vi "总磷总氮通讯.vi"() -> ()   [LabVIEW 2022 SP3, in "斯坦道CODcr.lvlib"]
uses:
  <vilib>/Plasmionique/MB Master/MB_Master_Serial/MB_Master_Serial.lvclass
  C:/Program Files (x86)/National Instruments/LabVIEW 2022/vi.lib/Plasmionique/MB Master/MB_Master/MB_Master.lvclass
  <vilib>/Plasmionique/MB Master/MB_Master_TCP/MB_Master_TCP.lvclass
  <vilib>/Utility/config.llb/Write Key (Boolean).vi
  <vilib>/Utility/config.llb/Write Key (String).vi
  <vilib>/Plasmionique/MB Master/MB_Master/MB_Master.lvclass
  <vilib>/Utility/config.llb/NI_LVConfig.lvlib
  <vilib>/Plasmionique/MB Master/MB Master.lvlib
  <vilib>/ptbypt/NI_PtbyPt.lvlib
panel:
  out "启用":bool=TRUE
  out "氨氮状态告警区":u16[](array[numeric])
  out "氨氮测量数据区":u16[](array[numeric])
  out "COD测量数据区":u16[](array[numeric])
  out "COD状态告警区":u16[](array[numeric])
  out "总氮测量数据区":u16[](array[numeric])
  out "总氮状态告警区":u16[](array[numeric])
  out "总磷状态告警区":u16[](array[numeric])
  out "总磷测量数据区":u16[](array[numeric])
  out "状态告警区":T1 {"告警代码" items=["无告警", "缺试剂告警", "缺水样告警", "缺蒸馏水告警", "缺标液告警", "仪表漏液告警", "标定异常告警", "超量程告警", "加热异常", "低试剂预警", "超上限告警", "超下限告警", "仪表内部其他异常", "滴定异常告警", "电极异常告警", "量程切换告警", "参数设置告警", "PH电极电位异常", "电导率电极异常", "浊度光度异常", "溶解氧电极异常", "溶解氧光强异常", "温度异常告警", "PH异常告警", "溶解氧异常告警", "电导率异常告警", "浊度异常告警", "叶绿素异常告警", "藻密度异常告警", "蓝绿藻异常告警", "ORP异常告警", "氨氮异常告警", "清洁刷异常告警", "SD卡异常告警", "蓝牙异常告警", "Wifi异常告警", "流程异常告警"]; "故障代码" items=["无故障", "电机故障", "温度故障", "通讯故障", "滴定故障"]}
  out "测量数据区":T2 {"单位" items=["ug/L", "mg/L", "ppm", "mg/m3", "cm", "ppb", "ug/m3", "%", "nmol/mol", "umol/mol", "MPN/L", "MPN/100ml", "ng/m3", "NTU", "无量纲", "ms/cm", "us/cm", "℃", "mV", "万个/L"]}
  out "status":bool
  out "关键参数区":T3
  in  "读关键参数区":bool
  in  "读状态告警区":bool
  in  "读测量数据区":bool
  in  "站号":u16(ring) items=["总磷"=1, "氨氮"=3]
  in  "停止":bool
  in  "启动":bool
  in  "控制命令":u16(ring) items=["启动测量"=1, "标样核查"=2, "零点核查"=3, "跨度核查"=4, "空白测试"=5, "平行样测试"=6, "加标回收"=7, "空白校准"=8, "标样校准"=9, "初始化（清洗）"=10, "停止测试"=11, "仪器重启"=12, "校时"=13, "模式设置"=14, "测量间隔设置"=15]
  in  "控制命令参数":u16[](array[numeric]) format="%04xH"
  in  "VISA Resource":refnum<visa-resource-name>
  in  "启用模块":bool
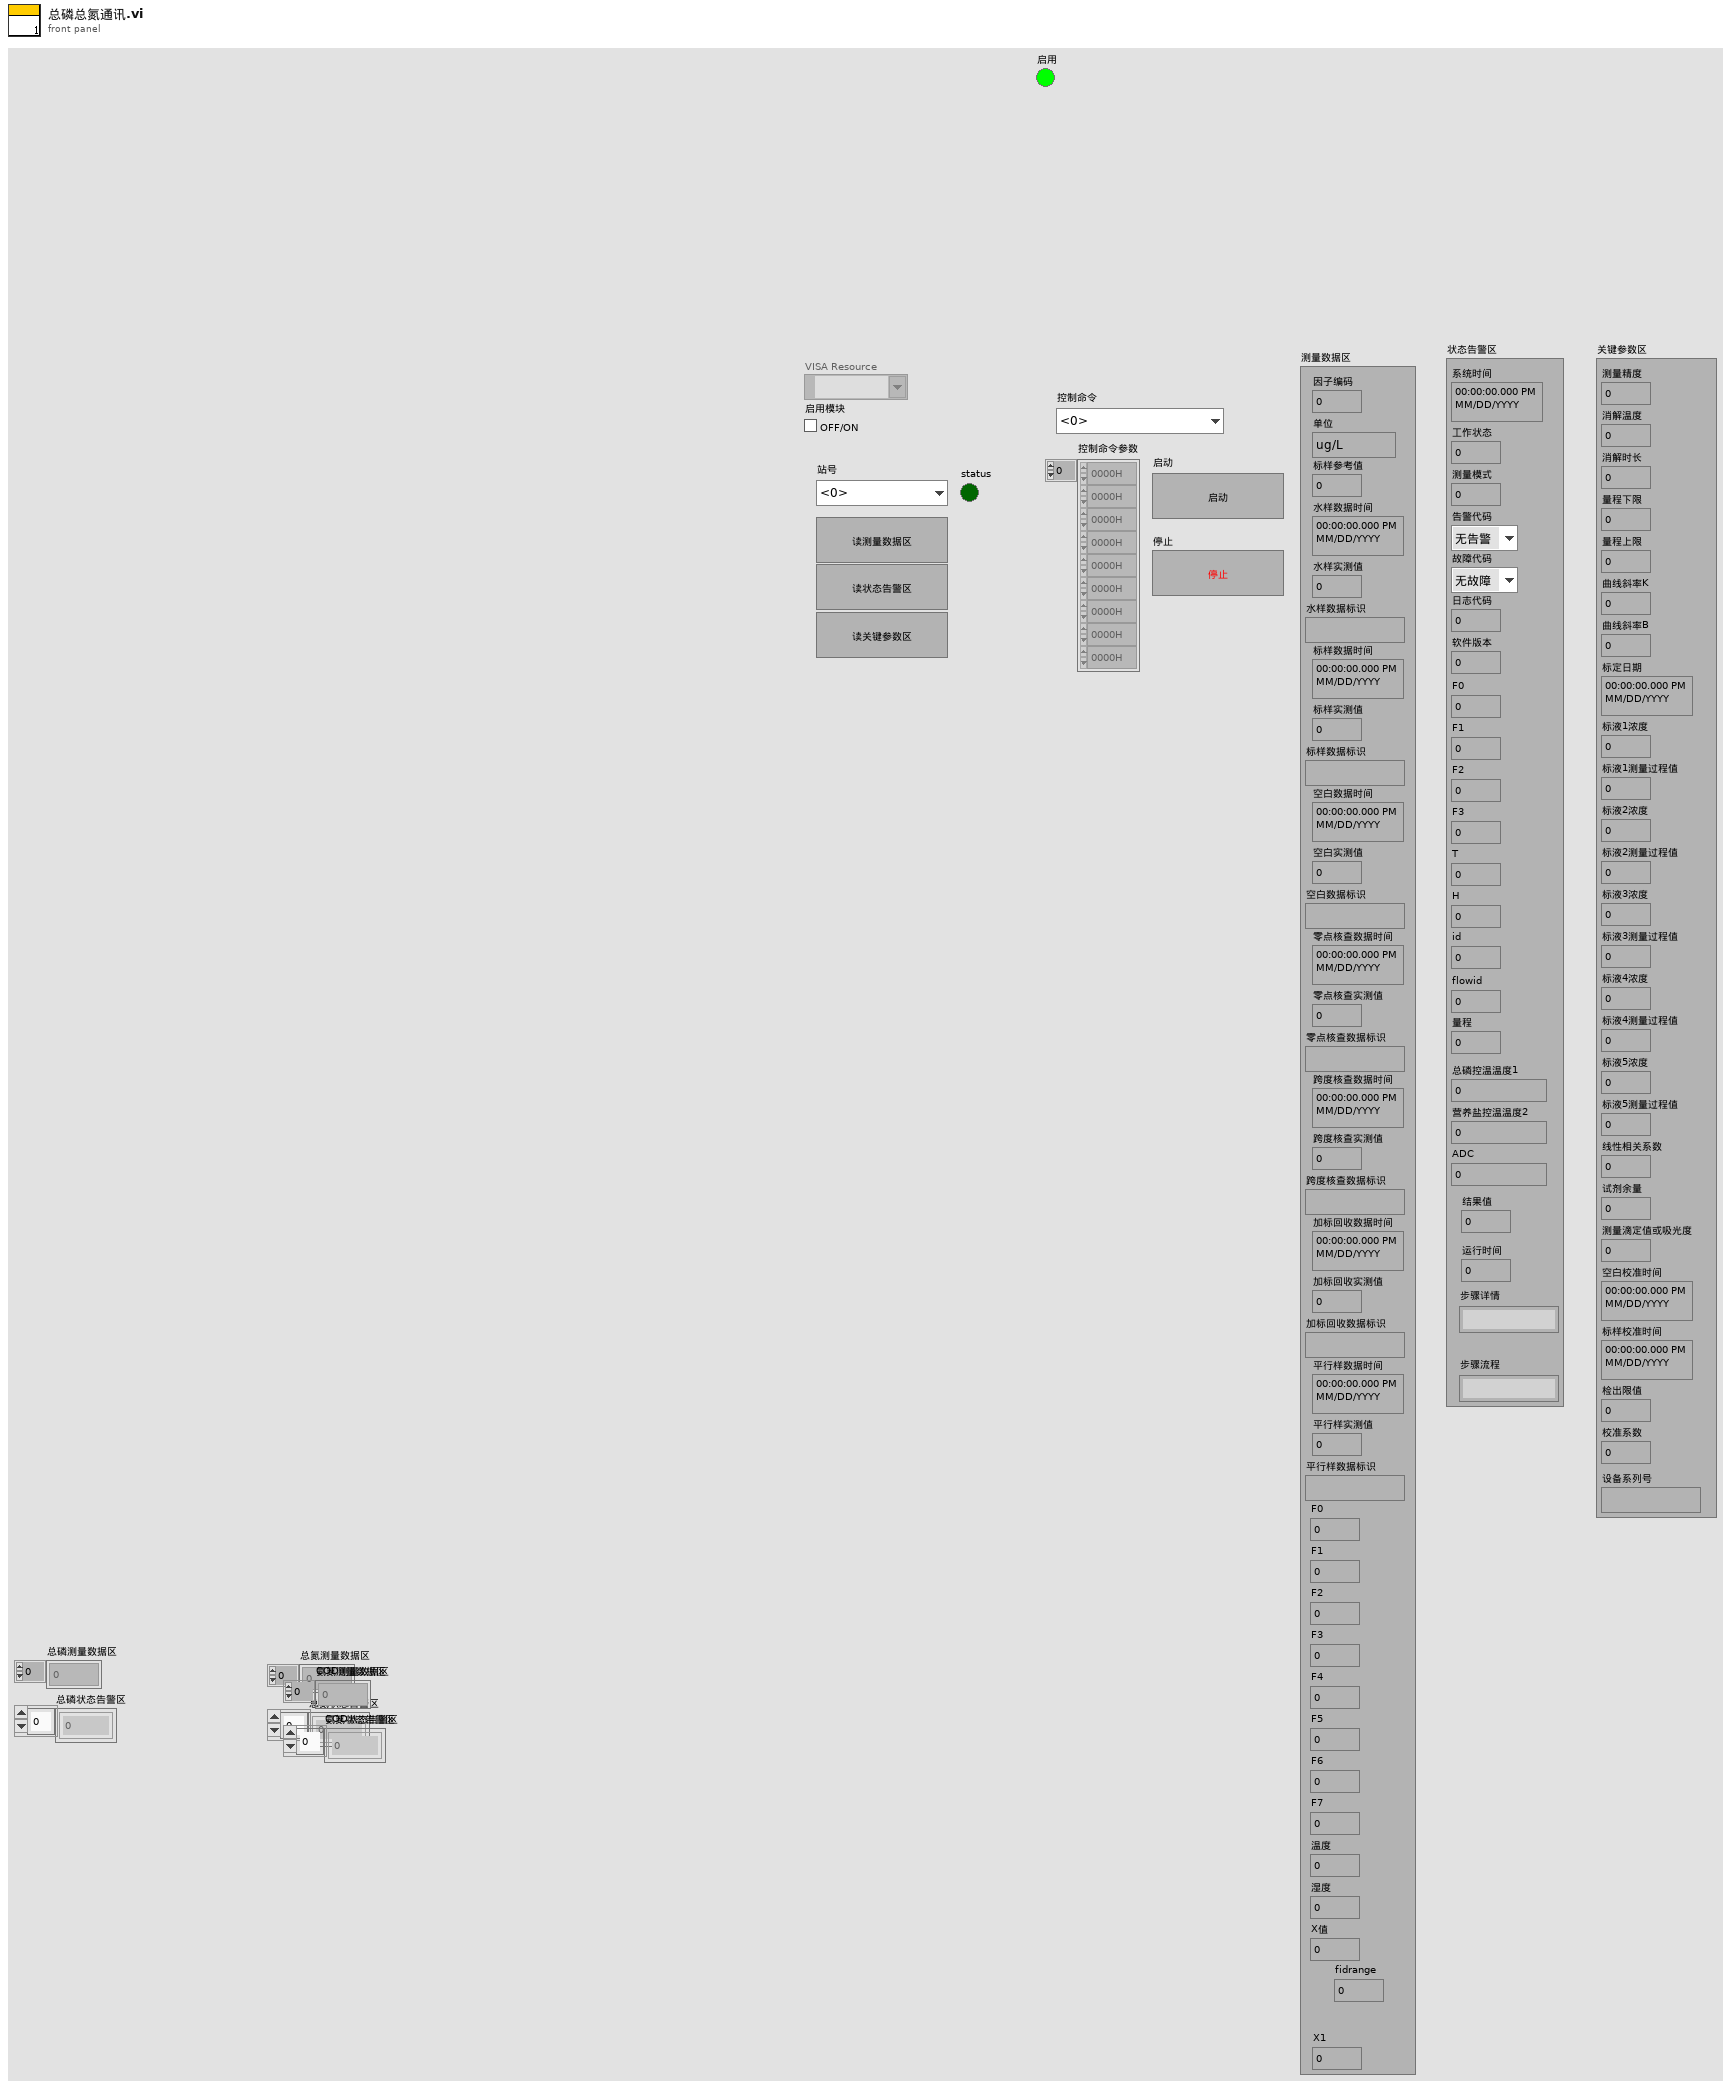
[diagram p1: front panel]
types:
  T1 = cluster{"系统时间":timestamp, "工作状态":u16, "测量模式":u16, "告警代码":u16, "故障代码":u16, "日志代码":u16, "软件版本":u16, "F0":sgl, "F1":sgl, "F2":sgl, "F3":sgl, "T":sgl, "H":sgl, "id":u16, "flowid":u16, "量程":u16, "总磷控温温度1":sgl, "营养盐控温温度2":sgl, "ADC":sgl, "结果值":sgl, "运行时间":u16, "步骤详情":string, "步骤流程":string}
  T2 = cluster{"因子编码":u32, "单位":u16, "标样参考值":sgl, "水样数据时间":timestamp, "水样实测值":sgl, "水样数据标识":string, "标样数据时间":timestamp, "标样实测值":sgl, "标样数据标识":string, "空白数据时间":timestamp, "空白实测值":sgl, "空白数据标识":string, "零点核查数据时间":timestamp, "零点核查实测值":sgl, "零点核查数据标识":string, "跨度核查数据时间":timestamp, "跨度核查实测值":sgl, "跨度核查数据标识":string, "加标回收数据时间":timestamp, "加标回收实测值":sgl, "加标回收数据标识":string, "平行样数据时间":timestamp, "平行样实测值":sgl, "平行样数据标识":string, "F0":sgl, "F1":sgl, "F2":sgl, "F3":sgl, "F4":sgl, "F5":sgl, "F6":sgl, "F7":sgl, "温度":sgl, "湿度":sgl, "X值":sgl, "fidrange":u16, "X1":sgl}
  T3 = cluster{"测量精度":u16, "消解温度":u16, "消解时长":u16, "量程下限":sgl, "量程上限":sgl, "曲线斜率K":sgl, "曲线斜率B":sgl, "标定日期":timestamp, "标液1浓度":sgl, "标液1测量过程值":sgl, "标液2浓度":sgl, "标液2测量过程值":sgl, "标液3浓度":sgl, "标液3测量过程值":sgl, "标液4浓度":sgl, "标液4测量过程值":sgl, "标液5浓度":sgl, "标液5测量过程值":sgl, "线性相关系数":sgl, "试剂余量":u32, "测量滴定值或吸光度":sgl, "空白校准时间":timestamp, "标样校准时间":timestamp, "检出限值":sgl, "校准系数":sgl, "设备系列号":string}
  T4 = cluster{"系统时间":timestamp, "工作状态":u16, "测量模式":enum16{"待机", "连续模式", "周期模式", "定点模式", "受控模式", "手动模式"}, "告警代码":u16, "故障代码":u16, "日志代码":u16, "软件版本":u16, "F0":sgl, "F1":sgl, "F2":sgl, "F3":sgl, "T":sgl, "H":sgl, "id":u16, "flowid":u16, "量程":u16, "总磷控温温度1":sgl, "营养盐控温温度2":sgl, "ADC":sgl}
  T5 = cluster{"因子编码":u32, "单位":u16, "标样参考值":sgl, "水样数据时间":timestamp, "水样实测值":sgl, "水样数据标识":string, "标样数据时间":timestamp, "标样实测值":sgl, "标样数据标识":string, "空白数据时间":timestamp, "空白实测值":sgl, "空白数据标识":string, "零点核查数据时间":timestamp, "零点核查实测值":sgl, "零点核查数据标识":string, "跨度核查数据时间":timestamp, "跨度核查实测值":sgl, "跨度核查数据标识":string, "加标回收数据时间":timestamp, "加标回收实测值":sgl, "加标回收数据标识":string, "平行样数据时间":timestamp, "平行样实测值":sgl, "平行样数据标识":string, "F0":sgl, "F1":sgl, "F2":sgl, "F3":sgl, "F4":sgl, "F5":sgl, "F6":sgl, "F7":sgl, "温度":sgl, "湿度":sgl, "X值":sgl, "fidrange":u16, "X1值":sgl}
  T6 = cluster{"测量精度":u16, "消解温度":u16, "消解时长":u16, "量程下限":sgl, "量程上限":sgl, "曲线斜率K":sgl, "曲线斜率B":sgl, "标定日期":timestamp, "标液1浓度":sgl, "标液1测量过程值":sgl, "标液2浓度":sgl, "标液2测量过程值":sgl, "标液3浓度":sgl, "标液3测量过程值":sgl, "标液4浓度":sgl, "标液4测量过程值":sgl, "标液5浓度":sgl, "标液5测量过程值":sgl, "线性相关系数":sgl, "试剂余量":u32, "测量滴定值或吸光度":sgl, "空白校准时间":timestamp, "标样校准时间":timestamp, "检出限值":sgl, "校准系数":sgl, "设备系列号":string}[]
  T7 = cluster{"系统时间":timestamp, "工作状态":u16, "测量模式":enum16{"待机", "连续模式", "周期模式", "定点模式", "受控模式", "手动模式"}, "告警代码":u16, "故障代码":u16, "日志代码":u16, "软件版本":u16, "F0":sgl, "F1":sgl, "F2":sgl, "F3":sgl, "T":sgl, "H":sgl, "id":u16, "flowid":u16, "量程":u16, "总磷控温温度1":sgl, "营养盐控温温度2":sgl, "ADC":sgl}[]
  T8 = cluster{"因子编码":u32, "单位":u16, "标样参考值":sgl, "水样数据时间":timestamp, "水样实测值":sgl, "水样数据标识":string, "标样数据时间":timestamp, "标样实测值":sgl, "标样数据标识":string, "空白数据时间":timestamp, "空白实测值":sgl, "空白数据标识":string, "零点核查数据时间":timestamp, "零点核查实测值":sgl, "零点核查数据标识":string, "跨度核查数据时间":timestamp, "跨度核查实测值":sgl, "跨度核查数据标识":string, "加标回收数据时间":timestamp, "加标回收实测值":sgl, "加标回收数据标识":string, "平行样数据时间":timestamp, "平行样实测值":sgl, "平行样数据标识":string, "F0":sgl, "F1":sgl, "F2":sgl, "F3":sgl, "F4":sgl, "F5":sgl, "F6":sgl, "F7":sgl, "温度":sgl, "湿度":sgl, "X值":sgl, "fidrange":u16, "X1值":sgl}[]
  T9 = enum16{"", "CODMn", "PH", "氨氮", "总氮", "总磷", "CODCr", "电导率", "水温", "溶解氧", "浊度", "叶绿素", "藻密度", "ORP"}
  T10 = typedef "CODCr交互.ctl" = cluster{"状态告警区":cluster{"系统时间":timestamp, "工作状态":u16, "测量模式":enum16{"待机", "连续模式", "周期模式", "定点模式", "受控模式", "手动模式"}, "告警代码":u16, "故障代码":u16, "日志代码":u16, "软件版本":u16, "F0":sgl, "F1":sgl, "F2":sgl, "F3":sgl, "T":sgl, "H":sgl, "id":u16, "flowid":u16, "量程":u16, "总磷控温温度1":sgl, "营养盐控温温度2":sgl, "ADC":sgl}, "平台试剂余量百分比":sgl, "关键参数":cluster{"测量量程":dbl, "测量精度":dbl, "测量间隔":dbl, "消解温度":dbl, "消解时长":dbl, "空白校准时间":timestamp, "曲线截距":dbl, "曲线斜率":dbl, "测量检出限":dbl, "测量信号值":dbl, "线性相关系数":dbl, "二次多项式系数":dbl, "标样校准时间":timestamp, "稀释倍数":dbl, "三项式系数":dbl, "空白标定系数":dbl, "量程系数":dbl, "F0/ORPA":dbl, "F1/ORPB":dbl, "F2/ORPK":dbl, "F3":dbl, "F4":dbl, "F5":dbl, "F6":dbl, "F7":dbl, "X0/滴定数":dbl, "量程":dbl}, "关键参数改变":bool, "校准信息":cluster{"低标液1浓度":dbl, "低标液1信号值":dbl, "低标液1启用":u16, "低标液2浓度":dbl, "低标液2信号值":dbl, "低标液2启用":u16, "低标液3浓度":dbl, "低标液3信号值":dbl, "低标液3启用":u16, "低标液4浓度":dbl, "低标液4信号值":dbl, "低标液4启用":u16, "低标液5浓度":dbl, "低标液5信号值":dbl, "低标液5启用":u16, "高标液1浓度":dbl, "高标液1信号值":dbl, "高标液1启用":u16, "高标液2浓度":dbl, "高标液2信号值":dbl, "高标液2启用":u16, "高标液3浓度":dbl, "高标液3信号值":dbl, "高标液3启用":u16, "高标液4浓度":dbl, "高标液4信号值":dbl, "高标液4启用":u16, "高标液5浓度":dbl, "高标液5信号值":dbl, "高标液5启用":u16, "低斜率":dbl, "低截距":dbl, "低二次多项式系数":dbl, "低线性相关系数":dbl, "高斜率":dbl, "高截距":dbl, "高二次多项式系数":dbl, "高线性相关系数":dbl}, "校准信息改变":bool, "固件版本号":string}
  T11 = typedef "总磷交互.ctl" = cluster{"状态告警区":cluster{"系统时间":timestamp, "工作状态":u16, "测量模式":enum16{"待机", "连续模式", "周期模式", "定点模式", "受控模式", "手动模式"}, "告警代码":u16, "故障代码":u16, "日志代码":u16, "软件版本":u16, "F0":sgl, "F1":sgl, "F2":sgl, "F3":sgl, "T":sgl, "H":sgl, "id":u16, "flowid":u16, "量程":u16, "总磷控温温度1":sgl, "营养盐控温温度2":sgl, "ADC":sgl}, "平台试剂余量百分比":sgl, "关键参数":cluster{"测量量程":dbl, "测量精度":dbl, "测量间隔":dbl, "消解温度":dbl, "消解时长":dbl, "空白校准时间":timestamp, "曲线截距":dbl, "曲线斜率":dbl, "测量检出限":dbl, "测量信号值":dbl, "线性相关系数":dbl, "二次多项式系数":dbl, "标样校准时间":timestamp, "稀释倍数":dbl, "三项式系数":dbl, "空白标定系数":dbl, "量程系数":dbl, "F0/ORPA":dbl, "F1/ORPB":dbl, "F2/ORPK":dbl, "F3":dbl, "F4":dbl, "F5":dbl, "F6":dbl, "F7":dbl, "X0/滴定数":dbl, "量程":dbl}, "关键参数改变":bool, "校准信息":cluster{"低标液1浓度":dbl, "低标液1信号值":dbl, "低标液1启用":u16, "低标液2浓度":dbl, "低标液2信号值":dbl, "低标液2启用":u16, "低标液3浓度":dbl, "低标液3信号值":dbl, "低标液3启用":u16, "低标液4浓度":dbl, "低标液4信号值":dbl, "低标液4启用":u16, "低标液5浓度":dbl, "低标液5信号值":dbl, "低标液5启用":u16, "高标液1浓度":dbl, "高标液1信号值":dbl, "高标液1启用":u16, "高标液2浓度":dbl, "高标液2信号值":dbl, "高标液2启用":u16, "高标液3浓度":dbl, "高标液3信号值":dbl, "高标液3启用":u16, "高标液4浓度":dbl, "高标液4信号值":dbl, "高标液4启用":u16, "高标液5浓度":dbl, "高标液5信号值":dbl, "高标液5启用":u16, "低斜率":dbl, "低截距":dbl, "低二次多项式系数":dbl, "低线性相关系数":dbl, "高斜率":dbl, "高截距":dbl, "高二次多项式系数":dbl, "高线性相关系数":dbl}, "校准信息改变":bool, "固件版本号":string}
  T12 = typedef "总氮交互.ctl" = cluster{"状态告警区":cluster{"系统时间":timestamp, "工作状态":u16, "测量模式":enum16{"待机", "连续模式", "周期模式", "定点模式", "受控模式", "手动模式"}, "告警代码":u16, "故障代码":u16, "日志代码":u16, "软件版本":u16, "F0":sgl, "F1":sgl, "F2":sgl, "F3":sgl, "T":sgl, "H":sgl, "id":u16, "flowid":u16, "量程":u16, "总磷控温温度1":sgl, "营养盐控温温度2":sgl, "ADC":sgl}, "平台试剂余量百分比":sgl, "关键参数":cluster{"测量量程":dbl, "测量精度":dbl, "测量间隔":dbl, "消解温度":dbl, "消解时长":dbl, "空白校准时间":timestamp, "曲线截距":dbl, "曲线斜率":dbl, "测量检出限":dbl, "测量信号值":dbl, "线性相关系数":dbl, "二次多项式系数":dbl, "标样校准时间":timestamp, "稀释倍数":dbl, "三项式系数":dbl, "空白标定系数":dbl, "量程系数":dbl, "F0/ORPA":dbl, "F1/ORPB":dbl, "F2/ORPK":dbl, "F3":dbl, "F4":dbl, "F5":dbl, "F6":dbl, "F7":dbl, "X0/滴定数":dbl, "量程":dbl}, "关键参数改变":bool, "校准信息":cluster{"低标液1浓度":dbl, "低标液1信号值":dbl, "低标液1启用":u16, "低标液2浓度":dbl, "低标液2信号值":dbl, "低标液2启用":u16, "低标液3浓度":dbl, "低标液3信号值":dbl, "低标液3启用":u16, "低标液4浓度":dbl, "低标液4信号值":dbl, "低标液4启用":u16, "低标液5浓度":dbl, "低标液5信号值":dbl, "低标液5启用":u16, "高标液1浓度":dbl, "高标液1信号值":dbl, "高标液1启用":u16, "高标液2浓度":dbl, "高标液2信号值":dbl, "高标液2启用":u16, "高标液3浓度":dbl, "高标液3信号值":dbl, "高标液3启用":u16, "高标液4浓度":dbl, "高标液4信号值":dbl, "高标液4启用":u16, "高标液5浓度":dbl, "高标液5信号值":dbl, "高标液5启用":u16, "低斜率":dbl, "低截距":dbl, "低二次多项式系数":dbl, "低线性相关系数":dbl, "高斜率":dbl, "高截距":dbl, "高二次多项式系数":dbl, "高线性相关系数":dbl}, "校准信息改变":bool, "固件版本号":string}
  T13 = typedef "氨氮交互.ctl" = cluster{"状态告警区":cluster{"系统时间":timestamp, "工作状态":u16, "测量模式":enum16{"待机", "连续模式", "周期模式", "定点模式", "受控模式", "手动模式"}, "告警代码":u16, "故障代码":u16, "日志代码":u16, "软件版本":u16, "F0":sgl, "F1":sgl, "F2":sgl, "F3":sgl, "T":sgl, "H":sgl, "id":u16, "flowid":u16, "量程":u16, "总磷控温温度1":sgl, "营养盐控温温度2":sgl, "ADC":sgl}, "平台试剂余量百分比":sgl, "关键参数":cluster{"测量量程":dbl, "测量精度":dbl, "测量间隔":dbl, "消解温度":dbl, "消解时长":dbl, "空白校准时间":timestamp, "曲线截距":dbl, "曲线斜率":dbl, "测量检出限":dbl, "测量信号值":dbl, "线性相关系数":dbl, "二次多项式系数":dbl, "标样校准时间":timestamp, "稀释倍数":dbl, "三项式系数":dbl, "空白标定系数":dbl, "量程系数":dbl, "F0/ORPA":dbl, "F1/ORPB":dbl, "F2/ORPK":dbl, "F3":dbl, "F4":dbl, "F5":dbl, "F6":dbl, "F7":dbl, "X0/滴定数":dbl, "量程":dbl}, "关键参数改变":bool, "校准信息":cluster{"低标液1浓度":dbl, "低标液1信号值":dbl, "低标液1启用":u16, "低标液2浓度":dbl, "低标液2信号值":dbl, "低标液2启用":u16, "低标液3浓度":dbl, "低标液3信号值":dbl, "低标液3启用":u16, "低标液4浓度":dbl, "低标液4信号值":dbl, "低标液4启用":u16, "低标液5浓度":dbl, "低标液5信号值":dbl, "低标液5启用":u16, "高标液1浓度":dbl, "高标液1信号值":dbl, "高标液1启用":u16, "高标液2浓度":dbl, "高标液2信号值":dbl, "高标液2启用":u16, "高标液3浓度":dbl, "高标液3信号值":dbl, "高标液3启用":u16, "高标液4浓度":dbl, "高标液4信号值":dbl, "高标液4启用":u16, "高标液5浓度":dbl, "高标液5信号值":dbl, "高标液5启用":u16, "低斜率":dbl, "低截距":dbl, "低二次多项式系数":dbl, "低线性相关系数":dbl, "高斜率":dbl, "高截距":dbl, "高二次多项式系数":dbl, "高线性相关系数":dbl}, "校准信息改变":bool, "固件版本号":string}
  T14 = typedef "NI_LVConfig.lvlib/Config Data RefNum.ctl" = refnum<k1>
  T15 = enum8{"Enabled", "Disabled", "Disabled and Grayed Out"}
  T16 = cluster{"baud rate (bps)":u32, "stop bits":u16, "parity":u16, "flow control":u16, "timeout":u32, "retries":i32}
  T17 = typedef "工况数据.ctl" = cluster{"time":string, "data":cluster{"ups":cluster{"ups":cluster{"input_voltage":ext, "input_frequency":ext, "output_voltage":ext, "output_current":ext, "output_frequency":ext, "output_active_power":ext, "output_apparent_power":ext, "load_rate":ext, "cabinet_temperature":ext, "battery_voltage":ext, "remaining_battery_capacity":ext, "power_on_status":string, "power_supply_mode":string, "fault":bool, "battery_low_voltage":bool, "mains_supply_abnormality":bool}, "启用":bool}, "air_conditioner":cluster{"air_conditioner":cluster{"cabinet_temperature":ext, "air_supply_temperature":ext, "voltage":ext, "current":ext, "compressor_status":string, "Internal_fan_status":string, "external_fan_status":string, "heating_state":string, "refrigeration_state":bool, "high_temperature_alarm":bool, "low_temperature_alarm":bool, "heater_fault":bool, "temperature_sensor_fault":bool, "high_voltage_alarm":bool, "low_voltage_alarm":bool, "refrigeration_start_point":ext, "refrigeration_sensitive_point":ext, "heating_start_point":ext, "heating_sensitive_point":ext, "high_temperature_alarm_point":ext, "low_temperature_alarm_point":ext}, "启用":bool}, "smoke_sensor":cluster{"smoke_sensor":cluster{"trigger_alarm":bool}, "启用":bool}, "water_immersion_sensor":cluster{"water_immersion_sensor":cluster{"trigger_alarm":bool}, "启用":bool}, "temperature_and_humidity_sensor":cluster{"temperature_and_humidity_sensor":cluster{"current_temperature":ext, "current_humidity":ext, "room_temperature_alarm":bool, "humidity_alarm":bool}, "启用":bool}, "gps":cluster{"gps":cluster{"current_longitude":ext, "current_latitude":ext, "launch_longitude":ext, "launch_latitude":ext, "shift_alarm":bool}, "启用":bool}, "solar_controller":cluster{"solar_controller":cluster{"array_voltage":ext, "array_current":ext, "generating_power":ext, "battery_voltage":dbl, "battery_current":ext, "ceiling_voltage":ext, "minimum_voltage":ext, "battery_temperature":ext, "remaining_battery_capacity":ext, "load_voltage":ext, "load_current":ext, "load_power":ext, "equipment_temperature":ext, "accumulated_electricity_consumption_of_the_day":ext, "accumulated_electricity_consumption_of_the_current_month":ext, "accumulated_electricity_consumption_in_the_current_year":ext, "total_accumulated_power_consumption":ext, "accumulated_charging_capacity_of_the_day":ext, "accumulated_charging_amount_of_the_current_month":ext, "accumulated_charging_capacity_of_the_current_year":ext, "total_cumulative_charge":ext}, "启用":bool}, "solar_controller_2":cluster{"solar_controller_2":cluster{"array_voltage":ext, "array_current":ext, "generating_power":ext, "battery_voltage":dbl, "battery_current":ext, "ceiling_voltage":ext, "minimum_voltage":ext, "battery_temperature":ext, "remaining_battery_capacity":ext, "load_voltage":ext, "load_current":ext, "load_power":ext, "equipment_temperature":ext, "accumulated_electricity_consumption_of_the_day":ext, "accumulated_electricity_consumption_of_the_current_month":ext, "accumulated_electricity_consumption_in_the_current_year":ext, "total_accumulated_power_consumption":ext, "accumulated_charging_capacity_of_the_day":ext, "accumulated_charging_amount_of_the_current_month":ext, "accumulated_charging_capacity_of_the_current_year":ext, "total_cumulative_charge":ext}, "启用":bool}, "NH3":cluster{"NH3":cluster{"F0":ext, "F1":ext, "syringe_temperature":ext, "alarm_step":dbl, "X0":ext}, "启用":bool}, "TP":cluster{"TP":cluster{"F0":ext, "F1":ext, "F2":ext, "F3":ext, "digestion_temperature":ext, "constant_temperature":ext, "syringe_temperature":ext, "alarm_step":dbl, "X0":ext}, "启用":bool}, "TN":cluster{"TN":cluster{"F0":ext, "F1":ext, "F2":ext, "F3":ext, "F4":ext, "F5":ext, "F6":ext, "F7":ext, "digestion_temperature":ext, "constant_temperature":ext, "syringe_temperature":ext, "alarm_step":dbl, "X0":ext}, "启用":bool}, "CODMn":cluster{"CODMn":cluster{"temperature_curve":ext[], "titration_curve":ext[], "F0":ext, "F1":ext, "F2":ext, "F3":ext, "F4":ext, "F5":ext, "A":ext, "B":ext, "K":ext}, "启用":bool}, "CODCr":cluster{"CODCr":cluster{"temperature_curve":ext[], "F0":ext, "F1":ext, "reagent_sensor":ext}, "启用":bool}}}
  T18 = cluster{"系统时间":timestamp, "工作状态":u16, "测量模式":enum16{"待机", "连续模式", "周期模式", "定点模式", "受控模式", "手动模式"}, "告警代码":u16, "故障代码":u16, "日志代码":u16, "软件版本":u16, "F0":sgl, "F1":sgl, "F2":sgl, "F3":sgl, "T":sgl, "H":sgl, "id":u16, "flowid":u16, "量程":u16, "总磷控温温度1":sgl, "营养盐控温温度2":sgl, "ADC":sgl, "结果值":sgl, "运行时间":u16, "步骤详情":string, "步骤流程":string}
  T19 = typedef "斯坦道CODcr.lvlib/关键参数.ctl" = cluster{"测量量程":sgl, "测量检出限":sgl, "测量精度":sgl, "测量间隔":sgl, "消解温度":sgl, "消解时长":sgl, "三项式系数":sgl, "二次多项式系数":sgl, "曲线斜率":sgl, "曲线截距":sgl, "线性相关系数":sgl, "空白校准时间":timestamp, "标样校准时间":timestamp, "测量信号值":sgl, "稀释倍数":sgl, "空白标定系数":sgl, "量程系数":sgl}
  T20 = cluster{"测量量程":dbl, "测量精度":dbl, "测量间隔":dbl, "消解温度":dbl, "消解时长":dbl, "空白校准时间":timestamp, "曲线截距":dbl, "曲线斜率":dbl, "测量检出限":dbl, "测量信号值":dbl, "线性相关系数":dbl, "二次多项式系数":dbl, "标样校准时间":timestamp, "稀释倍数":dbl, "三项式系数":dbl, "空白标定系数":dbl, "量程系数":dbl, "F0/ORPA":dbl, "F1/ORPB":dbl, "F2/ORPK":dbl, "F3":dbl, "F4":dbl, "F5":dbl, "F6":dbl, "F7":dbl, "X0/滴定数":dbl, "量程":dbl}
  T21 = cluster{"低标液1浓度":dbl, "低标液1信号值":dbl, "低标液1启用":u16, "低标液2浓度":dbl, "低标液2信号值":dbl, "低标液2启用":u16, "低标液3浓度":dbl, "低标液3信号值":dbl, "低标液3启用":u16, "低标液4浓度":dbl, "低标液4信号值":dbl, "低标液4启用":u16, "低标液5浓度":dbl, "低标液5信号值":dbl, "低标液5启用":u16, "高标液1浓度":dbl, "高标液1信号值":dbl, "高标液1启用":u16, "高标液2浓度":dbl, "高标液2信号值":dbl, "高标液2启用":u16, "高标液3浓度":dbl, "高标液3信号值":dbl, "高标液3启用":u16, "高标液4浓度":dbl, "高标液4信号值":dbl, "高标液4启用":u16, "高标液5浓度":dbl, "高标液5信号值":dbl, "高标液5启用":u16, "低斜率":dbl, "低截距":dbl, "低二次多项式系数":dbl, "低线性相关系数":dbl, "高斜率":dbl, "高截距":dbl, "高二次多项式系数":dbl, "高线性相关系数":dbl}
  T22 = typedef "操作日志字段定义.ctl" = cluster{"时间":timestamp, "参数":string, "日志信息":string, "流程参数":string}
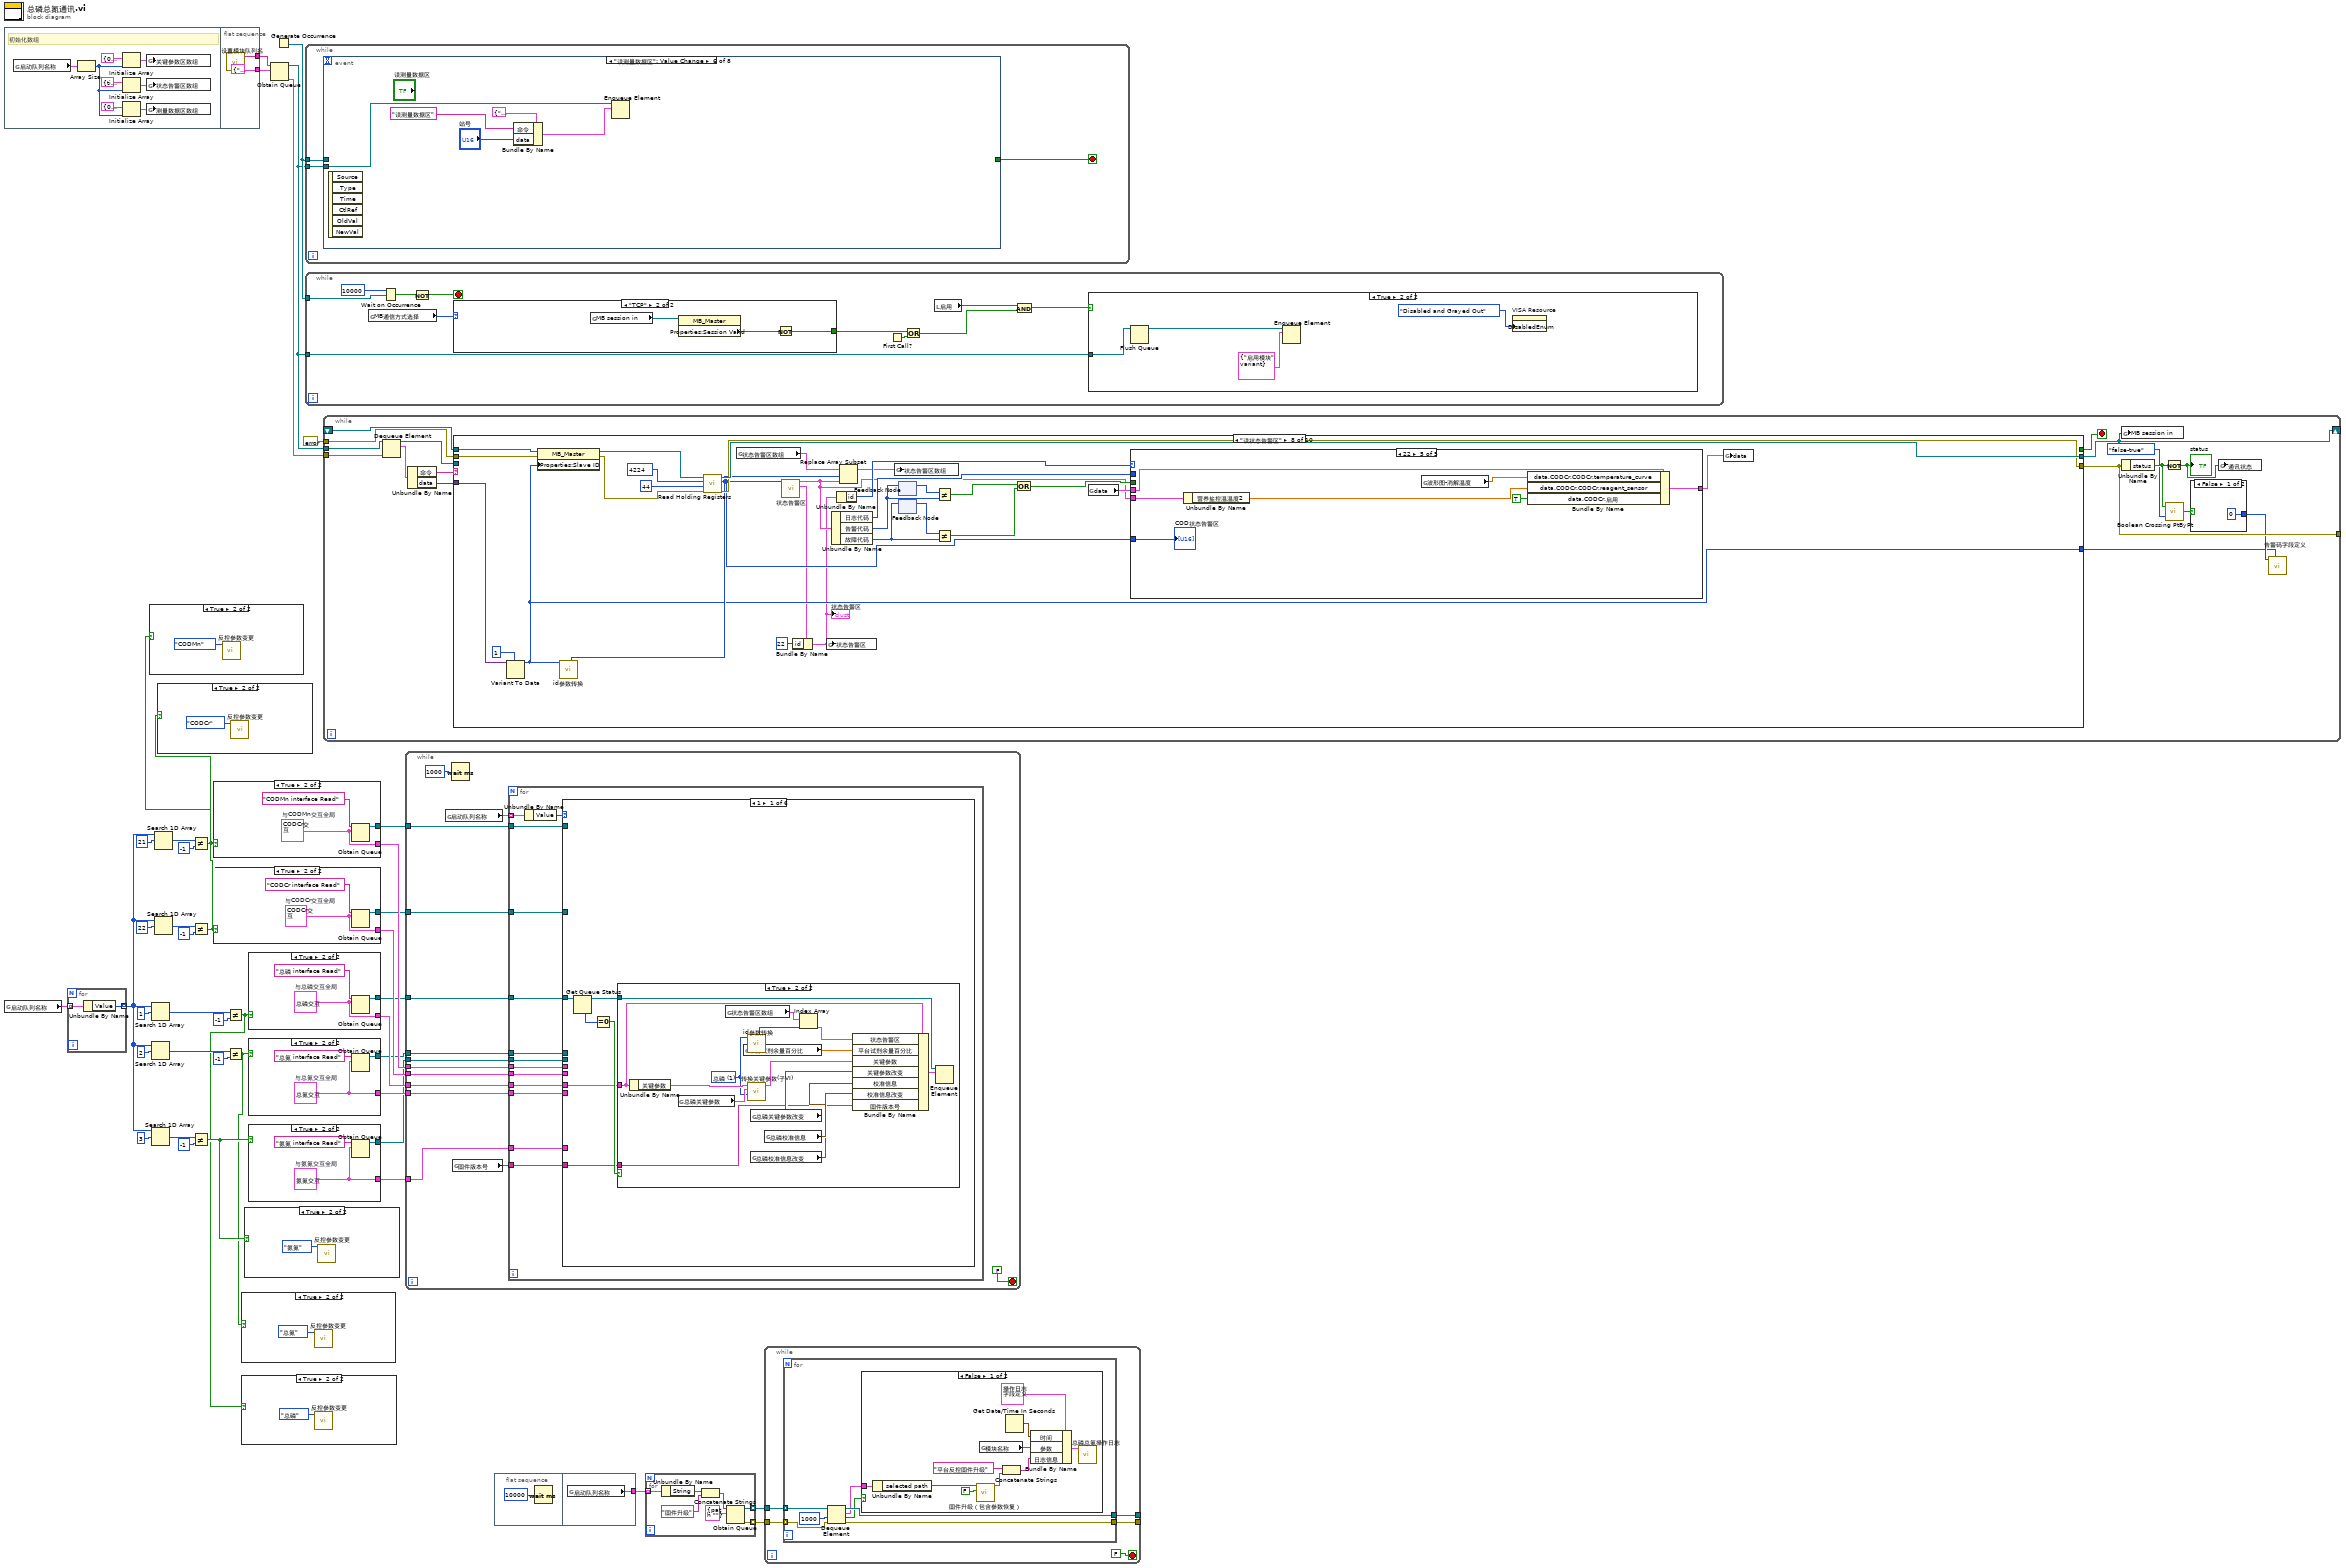
[diagram p0: block diagram]
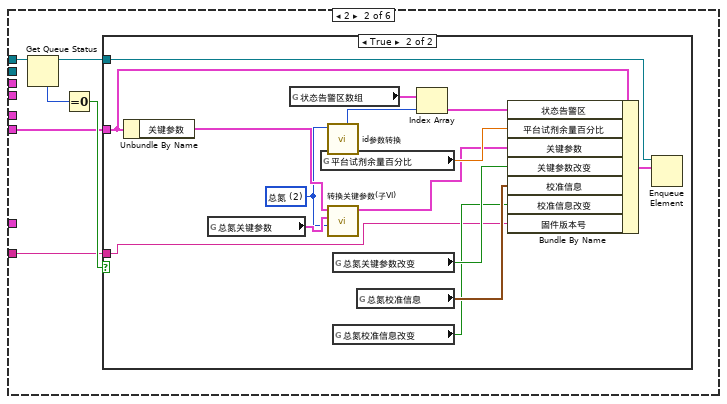
[diagram p14: hidden frame]
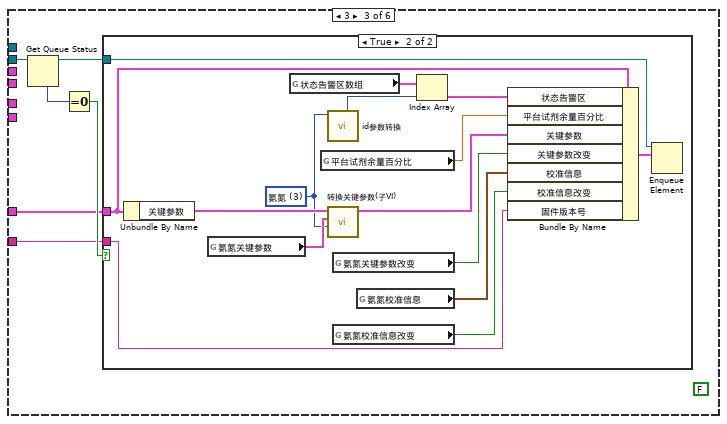
[diagram p16: hidden frame]
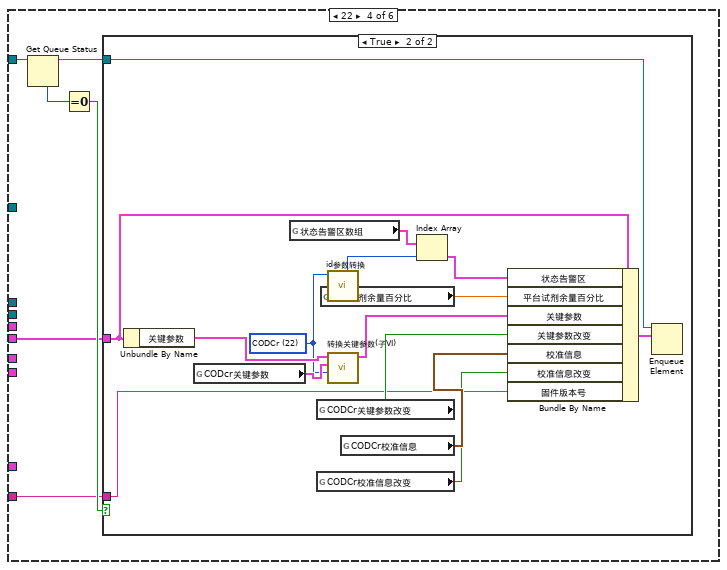
[diagram p18: hidden frame]
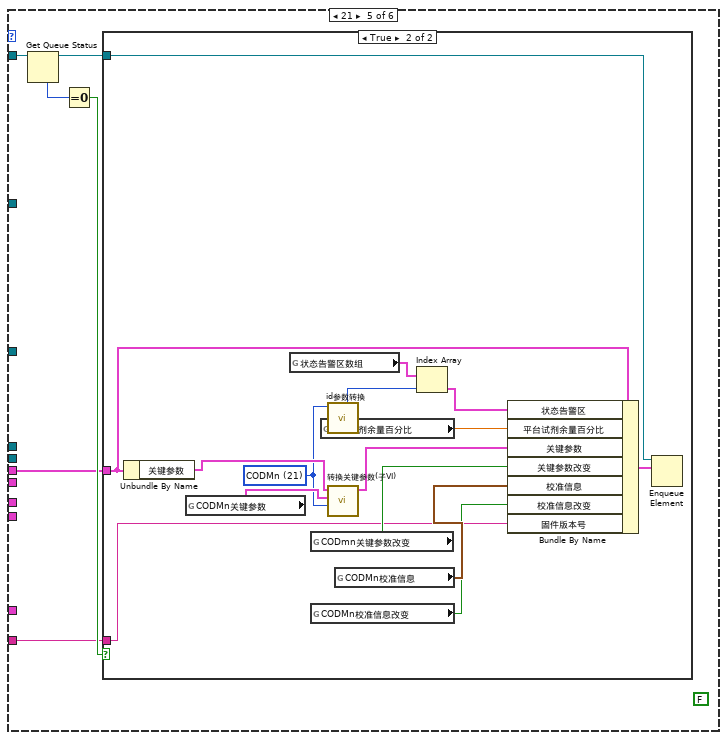
[diagram p20: hidden frame]
diagram:
  n1 = flat-sequence {
    tunnel: [cluster{"命令":string, "data":variant} {"命令"="", "data"=variant}] -> w41
    tunnel: [w50] -> w36
    frame #0 {
      # "初始化数组"
      n2 = global read "model config var.vi" "启动队列名称"() -> (w43:cluster{"String":string, "Value":u16}[])
      n3 = Array Size(array=w43) -> (size(s)=w42:i32)
      n4 = Initialize Array(T3 {"测量精度"=0, "消解温度"=0, "消解时长"=0, "量程下限"=0.0, "量程上限"=0.0, "曲线斜率K"=0.0, "曲线斜率B"=0.0, "标定日期"=timestamp(0 s since 1904-01-01), "标液1浓度"=0.0, "标液1测量过程值"=0.0, "标液2浓度"=0.0, "标液2测量过程值"=0.0, "标液3浓度"=0.0, "标液3测量过程值"=0.0, "标液4浓度"=0.0, "标液4测量过程值"=0.0, "标液5浓度"=0.0, "标液5测量过程值"=0.0, "线性相关系数"=0.0, "试剂余量"=0, "测量滴定值或吸光度"=0.0, "空白校准时间"=timestamp(0 s since 1904-01-01), "标样校准时间"=timestamp(0 s since 1904-01-01), "检出限值"=0.0, "校准系数"=0.0, "设备系列号"=""} ("关键参数区"), w42) -> (w47:T6)
      n5 = Initialize Array(T4 {"系统时间"=timestamp(0 s since 1904-01-01), "工作状态"=0, "测量模式"=enum."待机", "告警代码"=0, "故障代码"=0, "日志代码"=0, "软件版本"=0, "F0"=0.0, "F1"=0.0, "F2"=0.0, "F3"=0.0, "T"=0.0, "H"=0.0, "id"=0, "flowid"=0, "量程"=0, "总磷控温温度1"=0.0, "营养盐控温温度2"=0.0, "ADC"=0.0} ("状态告警区"), w42) -> (w46:T7)
      n6 = Initialize Array(T5 {"因子编码"=0, "单位"=0, "标样参考值"=0.0, "水样数据时间"=timestamp(0 s since 1904-01-01), "水样实测值"=0.0, "水样数据标识"="", "标样数据时间"=timestamp(0 s since 1904-01-01), "标样实测值"=0.0, "标样数据标识"="", "空白数据时间"=timestamp(0 s since 1904-01-01), "空白实测值"=0.0, "空白数据标识"="", "零点核查数据时间"=timestamp(0 s since 1904-01-01), "零点核查实测值"=0.0, "零点核查数据标识"="", "跨度核查数据时间"=timestamp(0 s since 1904-01-01), "跨度核查实测值"=0.0, "跨度核查数据标识"="", "加标回收数据时间"=timestamp(0 s since 1904-01-01), "加标回收实测值"=0.0, "加标回收数据标识"="", "平行样数据时间"=timestamp(0 s since 1904-01-01), "平行样实测值"=0.0, "平行样数据标识"="", "F0"=0.0, "F1"=0.0, "F2"=0.0, "F3"=0.0, "F4"=0.0, "F5"=0.0, "F6"=0.0, "F7"=0.0, "温度"=0.0, "湿度"=0.0, "X值"=0.0, "fidrange"=0, "X1值"=0.0} ("测量数据区"), w42) -> (w49:T8)
      n7 = global write "VAR总磷总氮全局变量.vi" "关键参数区数组"(w47) -> ()
      n8 = global write "VAR总磷总氮全局变量.vi" "状态告警区数组"(w46) -> ()
      n9 = global write "VAR总磷总氮全局变量.vi" "测量数据区数组"(w49) -> ()
    }
    frame #1 {
      n10 = call "设置模块队列名.vi"() -> ("Msg"=w50:string)  [unwired: 5 in]
    }
  }
  n11 = global read "model config var.vi" "启动队列名称"() -> (w25:cluster{"String":string, "Value":u16}[])
  n12 = for {
    tunnel: w25 -> [w53] mode=indexing
    tunnel: [w52] -> w9 mode=indexing
    n13 = Unbundle By Name(w53) -> ("Value"=w52:u16)
  }
  n14 = Search 1D Array(1D array=w9, element=u16 1 ("元素")) -> (index of element=w17:i32)  [unwired: 1 in]
  n15 = Search 1D Array(1D array=w9, element=u16 2 ("元素")) -> (index of element=w14:i32)  [unwired: 1 in]
  n16 = Search 1D Array(1D array=w9, element=u16 3 ("元素")) -> (index of element=w11:i32)  [unwired: 1 in]
  n17 = Search 1D Array(1D array=w9, element=u16 21 ("元素")) -> (index of element=w23:i32)  [unwired: 1 in]
  n18 = Search 1D Array(1D array=w9, element=u16 22 ("元素")) -> (index of element=w20:i32)  [unwired: 1 in]
  n19 = Not Equal?(x=w23, y=-1) -> (x != y?=w1:bool)
  n20 = case shown="True" w1 {
    frame False {
    }
    frame True {
      n21 = call "反控参数变更.vi"("设置参数"=T9."CODMn") -> ()  [unwired: 11 in]
    }
  }
  n22 = Not Equal?(x=w20, y=-1) -> (x != y?=w2:bool)
  n23 = case shown="True" w2 {
    frame False {
    }
    frame True {
      n24 = call "反控参数变更.vi"("设置参数"=T9."CODCr") -> ()  [unwired: 11 in]
    }
  }
  n25 = Not Equal?(x=w11, y=-1) -> (x != y?=w5:bool)
  n26 = case shown="True" w1 {
    tunnel: [_ w57] -> w35
    tunnel: [_ w56] -> w34
    frame False {
    }
    frame True {
      w56 = T10 {"状态告警区"={"系统时间"=timestamp(0 s since 1904-01-01), "工作状态"=0, "测量模式"=enum."待机", "告警代码"=0, "故障代码"=0, "日志代码"=0, "软件版本"=0, "F0"=0.0, "F1"=0.0, "F2"=0.0, "F3"=0.0, "T"=0.0, "H"=0.0, "id"=0, "flowid"=0, "量程"=0, "总磷控温温度1"=0.0, "营养盐控温温度2"=0.0, "ADC"=0.0}, "平台试剂余量百分比"=0.0, "关键参数"={"测量量程"=0.0, "测量精度"=0.0, "测量间隔"=0.0, "消解温度"=0.0, "消解时长"=0.0, "空白校准时间"=timestamp(0 s since 1904-01-01), "曲线截距"=0.0, "曲线斜率"=0.0, "测量检出限"=0.0, "测量信号值"=0.0, "线性相关系数"=0.0, "二次多项式系数"=0.0, "标样校准时间"=timestamp(0 s since 1904-01-01), "稀释倍数"=0.0, "三项式系数"=0.0, "空白标定系数"=0.0, "量程系数"=0.0, "F0/ORPA"=0.0, "F1/ORPB"=0.0, "F2/ORPK"=0.0, "F3"=0.0, "F4"=0.0, "F5"=0.0, "F6"=0.0, "F7"=0.0, "X0/滴定数"=0.0, "量程"=0.0}, "关键参数改变"=FALSE, "校准信息"={"低标液1浓度"=0.0, "低标液1信号值"=0.0, "低标液1启用"=0, "低标液2浓度"=0.0, "低标液2信号值"=0.0, "低标液2启用"=0, "低标液3浓度"=0.0, "低标液3信号值"=0.0, "低标液3启用"=0, "低标液4浓度"=0.0, "低标液4信号值"=0.0, "低标液4启用"=0, "低标液5浓度"=0.0, "低标液5信号值"=0.0, "低标液5启用"=0, "高标液1浓度"=0.0, "高标液1信号值"=0.0, "高标液1启用"=0, "高标液2浓度"=0.0, "高标液2信号值"=0.0, "高标液2启用"=0, "高标液3浓度"=0.0, "高标液3信号值"=0.0, "高标液3启用"=0, "高标液4浓度"=0.0, "高标液4信号值"=0.0, "高标液4启用"=0, "高标液5浓度"=0.0, "高标液5信号值"=0.0, "高标液5启用"=0, "低斜率"=0.0, "低截距"=0.0, "低二次多项式系数"=0.0, "低线性相关系数"=0.0, "高斜率"=0.0, "高截距"=0.0, "高二次多项式系数"=0.0, "高线性相关系数"=0.0}, "校准信息改变"=FALSE, "固件版本号"=""}  # 与CODMn交互全局
      n27 = Obtain Queue(name (unnamed)="CODMn interface Read" ("写入方名称"), element data type=w56) -> (queue out=w57:refnum<queue>)  [unwired: 3 in, 2 out]
    }
  }
  n28 = case shown="True" w2 {
    tunnel: [_ w60] -> w33
    tunnel: [_ w59] -> w32
    frame False {
    }
    frame True {
      w59 = T10 {"状态告警区"={"系统时间"=timestamp(0 s since 1904-01-01), "工作状态"=0, "测量模式"=enum."待机", "告警代码"=0, "故障代码"=0, "日志代码"=0, "软件版本"=0, "F0"=0.0, "F1"=0.0, "F2"=0.0, "F3"=0.0, "T"=0.0, "H"=0.0, "id"=0, "flowid"=0, "量程"=0, "总磷控温温度1"=0.0, "营养盐控温温度2"=0.0, "ADC"=0.0}, "平台试剂余量百分比"=0.0, "关键参数"={"测量量程"=0.0, "测量精度"=0.0, "测量间隔"=0.0, "消解温度"=0.0, "消解时长"=0.0, "空白校准时间"=timestamp(0 s since 1904-01-01), "曲线截距"=0.0, "曲线斜率"=0.0, "测量检出限"=0.0, "测量信号值"=0.0, "线性相关系数"=0.0, "二次多项式系数"=0.0, "标样校准时间"=timestamp(0 s since 1904-01-01), "稀释倍数"=0.0, "三项式系数"=0.0, "空白标定系数"=0.0, "量程系数"=0.0, "F0/ORPA"=0.0, "F1/ORPB"=0.0, "F2/ORPK"=0.0, "F3"=0.0, "F4"=0.0, "F5"=0.0, "F6"=0.0, "F7"=0.0, "X0/滴定数"=0.0, "量程"=0.0}, "关键参数改变"=FALSE, "校准信息"={"低标液1浓度"=0.0, "低标液1信号值"=0.0, "低标液1启用"=0, "低标液2浓度"=0.0, "低标液2信号值"=0.0, "低标液2启用"=0, "低标液3浓度"=0.0, "低标液3信号值"=0.0, "低标液3启用"=0, "低标液4浓度"=0.0, "低标液4信号值"=0.0, "低标液4启用"=0, "低标液5浓度"=0.0, "低标液5信号值"=0.0, "低标液5启用"=0, "高标液1浓度"=0.0, "高标液1信号值"=0.0, "高标液1启用"=0, "高标液2浓度"=0.0, "高标液2信号值"=0.0, "高标液2启用"=0, "高标液3浓度"=0.0, "高标液3信号值"=0.0, "高标液3启用"=0, "高标液4浓度"=0.0, "高标液4信号值"=0.0, "高标液4启用"=0, "高标液5浓度"=0.0, "高标液5信号值"=0.0, "高标液5启用"=0, "低斜率"=0.0, "低截距"=0.0, "低二次多项式系数"=0.0, "低线性相关系数"=0.0, "高斜率"=0.0, "高截距"=0.0, "高二次多项式系数"=0.0, "高线性相关系数"=0.0}, "校准信息改变"=FALSE, "固件版本号"=""}  # 与CODCr交互全局
      n29 = Obtain Queue(name (unnamed)="CODCr interface Read" ("写入方名称"), element data type=w59) -> (queue out=w60:refnum<queue>)  [unwired: 3 in, 2 out]
    }
  }
  n30 = Not Equal?(x=w17, y=-1) -> (x != y?=w3:bool)
  n31 = Not Equal?(x=w14, y=-1) -> (x != y?=w4:bool)
  n32 = case shown="True" w4 {
    frame False {
    }
    frame True {
      n33 = call "反控参数变更.vi"("设置参数"=T9."总氮") -> ()  [unwired: 11 in]
    }
  }
  n34 = case shown="True" w3 {
    frame False {
    }
    frame True {
      n35 = call "反控参数变更.vi"("设置参数"=T9."总磷") -> ()  [unwired: 11 in]
    }
  }
  n36 = case shown="True" w5 {
    frame False {
    }
    frame True {
      n37 = call "反控参数变更.vi"("设置参数"=T9."氨氮") -> ()  [unwired: 11 in]
    }
  }
  n38 = case shown="True" w3 {
    tunnel: [_ w66] -> w31
    tunnel: [_ w65] -> w30
    frame False {
    }
    frame True {
      w65 = T11 {"状态告警区"={"系统时间"=timestamp(0 s since 1904-01-01), "工作状态"=0, "测量模式"=enum."待机", "告警代码"=0, "故障代码"=0, "日志代码"=0, "软件版本"=0, "F0"=0.0, "F1"=0.0, "F2"=0.0, "F3"=0.0, "T"=0.0, "H"=0.0, "id"=0, "flowid"=0, "量程"=0, "总磷控温温度1"=0.0, "营养盐控温温度2"=0.0, "ADC"=0.0}, "平台试剂余量百分比"=0.0, "关键参数"={"测量量程"=0.0, "测量精度"=0.0, "测量间隔"=0.0, "消解温度"=0.0, "消解时长"=0.0, "空白校准时间"=timestamp(0 s since 1904-01-01), "曲线截距"=0.0, "曲线斜率"=0.0, "测量检出限"=0.0, "测量信号值"=0.0, "线性相关系数"=0.0, "二次多项式系数"=0.0, "标样校准时间"=timestamp(0 s since 1904-01-01), "稀释倍数"=0.0, "三项式系数"=0.0, "空白标定系数"=0.0, "量程系数"=0.0, "F0/ORPA"=0.0, "F1/ORPB"=0.0, "F2/ORPK"=0.0, "F3"=0.0, "F4"=0.0, "F5"=0.0, "F6"=0.0, "F7"=0.0, "X0/滴定数"=0.0, "量程"=0.0}, "关键参数改变"=FALSE, "校准信息"={"低标液1浓度"=0.0, "低标液1信号值"=0.0, "低标液1启用"=0, "低标液2浓度"=0.0, "低标液2信号值"=0.0, "低标液2启用"=0, "低标液3浓度"=0.0, "低标液3信号值"=0.0, "低标液3启用"=0, "低标液4浓度"=0.0, "低标液4信号值"=0.0, "低标液4启用"=0, "低标液5浓度"=0.0, "低标液5信号值"=0.0, "低标液5启用"=0, "高标液1浓度"=0.0, "高标液1信号值"=0.0, "高标液1启用"=0, "高标液2浓度"=0.0, "高标液2信号值"=0.0, "高标液2启用"=0, "高标液3浓度"=0.0, "高标液3信号值"=0.0, "高标液3启用"=0, "高标液4浓度"=0.0, "高标液4信号值"=0.0, "高标液4启用"=0, "高标液5浓度"=0.0, "高标液5信号值"=0.0, "高标液5启用"=0, "低斜率"=0.0, "低截距"=0.0, "低二次多项式系数"=0.0, "低线性相关系数"=0.0, "高斜率"=0.0, "高截距"=0.0, "高二次多项式系数"=0.0, "高线性相关系数"=0.0}, "校准信息改变"=FALSE, "固件版本号"=""}  # 与总磷交互全局
      n39 = Obtain Queue(name (unnamed)="总磷 interface Read" ("写入方名称"), element data type=w65) -> (queue out=w66:refnum<queue>)  [unwired: 3 in, 2 out]
    }
  }
  n40 = case shown="True" w4 {
    tunnel: [_ w69] -> w29
    tunnel: [_ w68] -> w28
    frame False {
    }
    frame True {
      w68 = T12 {"状态告警区"={"系统时间"=timestamp(0 s since 1904-01-01), "工作状态"=0, "测量模式"=enum."待机", "告警代码"=0, "故障代码"=0, "日志代码"=0, "软件版本"=0, "F0"=0.0, "F1"=0.0, "F2"=0.0, "F3"=0.0, "T"=0.0, "H"=0.0, "id"=0, "flowid"=0, "量程"=0, "总磷控温温度1"=0.0, "营养盐控温温度2"=0.0, "ADC"=0.0}, "平台试剂余量百分比"=0.0, "关键参数"={"测量量程"=0.0, "测量精度"=0.0, "测量间隔"=0.0, "消解温度"=0.0, "消解时长"=0.0, "空白校准时间"=timestamp(0 s since 1904-01-01), "曲线截距"=0.0, "曲线斜率"=0.0, "测量检出限"=0.0, "测量信号值"=0.0, "线性相关系数"=0.0, "二次多项式系数"=0.0, "标样校准时间"=timestamp(0 s since 1904-01-01), "稀释倍数"=0.0, "三项式系数"=0.0, "空白标定系数"=0.0, "量程系数"=0.0, "F0/ORPA"=0.0, "F1/ORPB"=0.0, "F2/ORPK"=0.0, "F3"=0.0, "F4"=0.0, "F5"=0.0, "F6"=0.0, "F7"=0.0, "X0/滴定数"=0.0, "量程"=0.0}, "关键参数改变"=FALSE, "校准信息"={"低标液1浓度"=0.0, "低标液1信号值"=0.0, "低标液1启用"=0, "低标液2浓度"=0.0, "低标液2信号值"=0.0, "低标液2启用"=0, "低标液3浓度"=0.0, "低标液3信号值"=0.0, "低标液3启用"=0, "低标液4浓度"=0.0, "低标液4信号值"=0.0, "低标液4启用"=0, "低标液5浓度"=0.0, "低标液5信号值"=0.0, "低标液5启用"=0, "高标液1浓度"=0.0, "高标液1信号值"=0.0, "高标液1启用"=0, "高标液2浓度"=0.0, "高标液2信号值"=0.0, "高标液2启用"=0, "高标液3浓度"=0.0, "高标液3信号值"=0.0, "高标液3启用"=0, "高标液4浓度"=0.0, "高标液4信号值"=0.0, "高标液4启用"=0, "高标液5浓度"=0.0, "高标液5信号值"=0.0, "高标液5启用"=0, "低斜率"=0.0, "低截距"=0.0, "低二次多项式系数"=0.0, "低线性相关系数"=0.0, "高斜率"=0.0, "高截距"=0.0, "高二次多项式系数"=0.0, "高线性相关系数"=0.0}, "校准信息改变"=FALSE, "固件版本号"=""}  # 与总氮交互全局
      n41 = Obtain Queue(name (unnamed)="总氮 interface Read" ("写入方名称"), element data type=w68) -> (queue out=w69:refnum<queue>)  [unwired: 3 in, 2 out]
    }
  }
  n42 = case shown="True" w5 {
    tunnel: [_ w72] -> w27
    tunnel: [_ w71] -> w26
    frame False {
    }
    frame True {
      w71 = T13 {"状态告警区"={"系统时间"=timestamp(0 s since 1904-01-01), "工作状态"=0, "测量模式"=enum."待机", "告警代码"=0, "故障代码"=0, "日志代码"=0, "软件版本"=0, "F0"=0.0, "F1"=0.0, "F2"=0.0, "F3"=0.0, "T"=0.0, "H"=0.0, "id"=0, "flowid"=0, "量程"=0, "总磷控温温度1"=0.0, "营养盐控温温度2"=0.0, "ADC"=0.0}, "平台试剂余量百分比"=0.0, "关键参数"={"测量量程"=0.0, "测量精度"=0.0, "测量间隔"=0.0, "消解温度"=0.0, "消解时长"=0.0, "空白校准时间"=timestamp(0 s since 1904-01-01), "曲线截距"=0.0, "曲线斜率"=0.0, "测量检出限"=0.0, "测量信号值"=0.0, "线性相关系数"=0.0, "二次多项式系数"=0.0, "标样校准时间"=timestamp(0 s since 1904-01-01), "稀释倍数"=0.0, "三项式系数"=0.0, "空白标定系数"=0.0, "量程系数"=0.0, "F0/ORPA"=0.0, "F1/ORPB"=0.0, "F2/ORPK"=0.0, "F3"=0.0, "F4"=0.0, "F5"=0.0, "F6"=0.0, "F7"=0.0, "X0/滴定数"=0.0, "量程"=0.0}, "关键参数改变"=FALSE, "校准信息"={"低标液1浓度"=0.0, "低标液1信号值"=0.0, "低标液1启用"=0, "低标液2浓度"=0.0, "低标液2信号值"=0.0, "低标液2启用"=0, "低标液3浓度"=0.0, "低标液3信号值"=0.0, "低标液3启用"=0, "低标液4浓度"=0.0, "低标液4信号值"=0.0, "低标液4启用"=0, "低标液5浓度"=0.0, "低标液5信号值"=0.0, "低标液5启用"=0, "高标液1浓度"=0.0, "高标液1信号值"=0.0, "高标液1启用"=0, "高标液2浓度"=0.0, "高标液2信号值"=0.0, "高标液2启用"=0, "高标液3浓度"=0.0, "高标液3信号值"=0.0, "高标液3启用"=0, "高标液4浓度"=0.0, "高标液4信号值"=0.0, "高标液4启用"=0, "高标液5浓度"=0.0, "高标液5信号值"=0.0, "高标液5启用"=0, "低斜率"=0.0, "低截距"=0.0, "低二次多项式系数"=0.0, "低线性相关系数"=0.0, "高斜率"=0.0, "高截距"=0.0, "高二次多项式系数"=0.0, "高线性相关系数"=0.0}, "校准信息改变"=FALSE, "固件版本号"=""}  # 与氨氮交互全局
      n43 = Obtain Queue(name (unnamed)="氨氮 interface Read" ("写入方名称"), element data type=w71) -> (queue out=w72:refnum<queue>)  [unwired: 3 in, 2 out]
    }
  }
  n44 = Obtain Queue(name (unnamed)=w36, element data type=w41) -> (queue out=w37:refnum<queue>, error out=w40:errorcluster)  [unwired: 3 in, 1 out]
  n45 = Generate Occurrence() -> (w38:refnum<k4>)
  n46 = while {
    tunnel: w37 -> [w76]
    tunnel: w38 -> [w74]
    stop <- w75 stop-if-true
    n47 = event shown="[5] \"读测量数据区\": Value Change" {
      selector: _ -> [_ _ _ _ _ _ _ _]
      dyn-events: _ -> [_ _ _ _ _ _ _ _]
      timeout: _ -> [_ _ _ _ _ _ _ _]
      tunnel: w76 -> [_ _ _ w108 w118 w124 w129 w134]
      tunnel: [_ _ _ _ "停止" _ _ _] -> w75
      tunnel: w74 -> [_ _ _ _ w115 _ _ _]
      event Timeout {
        n48 = event-data() -> ()  [unwired: 1 in, 3 out]
      }
      event "启用模块": Value Change {
        n49 = event-data() -> ("NewVal"=w77:bool)  [unwired: 1 in, 5 out]
        n50 = call <vilib>:"Application Directory.vi"() -> ("Application Directory"=w79:path)
        n51 = Build Path(base path=w79, name or relative path="data\\set.ini" ("名称或相对路径")) -> (appended path=w80:path)
        n52 = call <vilib>:"Open Config Data.vi"("configuration file path"=w80) -> ("error out"=w86:errorcluster, "refnum"=w85:T14)  [unwired: 8 in, 1 out]
        n53 = call-poly <vilib>:"Write Key.vi"("section"="总磷总氮", "error in (no error)"=w86, "value"=w77, "key"="模块启用", "refnum"=w85) -> ("error out"=w82:errorcluster, "refnum out"=w78:T14)  [unwired: 4 in, 1 out]
        n54 = call <vilib>:"Close Config Data.vi"("error in (no error)"=w82, "refnum"=w78) -> ()  [unwired: 8 in, 2 out]
      }
      event "VISA Resource": Value Change {
        n55 = event-data() -> ()  [unwired: 1 in, 6 out]
        n56 = call <vilib>:"Application Directory.vi"() -> ("Application Directory"=w89:path)
        n57 = Build Path(base path=w89, name or relative path="data\\set.ini" ("名称或相对路径")) -> (appended path=w90:path)
        n58 = call <vilib>:"Open Config Data.vi"("configuration file path"=w90) -> ("error out"=w96:errorcluster, "refnum"=w95:T14)  [unwired: 8 in, 1 out]
        n59 = call-poly <vilib>:"Write Key.vi"("section"="总磷总氮", "error in (no error)"=w96, "value"="VISA Resource", "key"="串口", "refnum"=w95) -> ("error out"=w92:errorcluster, "refnum out"=w88:T14)  [unwired: 4 in, 1 out]
        n60 = call <vilib>:"Close Config Data.vi"("error in (no error)"=w92, "refnum"=w88) -> ()  [unwired: 8 in, 2 out]
      }
      event "启动": Value Change {
        n61 = event-data() -> ()  [unwired: 1 in, 6 out]
        n62 = global read "总磷总氮断电保存全局变量.vi" "协议"() -> (w99:u16)
        n63 = case shown="Default" "控制命令" {
          tunnel: "控制命令参数" -> [w113 w114]
          tunnel: [w112 w114] -> w100
          frame Default {
            n64 = call "HexToWord.vi"("数组"=w113) -> ("WORD"=w112:u16[])  [unwired: 10 in]
          }
          frame 13 {
          }
        }
        n65 = case shown="1" w99 {
          tunnel: "控制命令" -> [w109 w111]
          tunnel: [w109 w110] -> w97
          frame 0, Default {
          }
          frame 1 {
            n66 = Swap Bytes(anything=w111) -> (byte swapped=w110:u16)
          }
        }
        n67 = call "控制命令区.vi"("控制命令参数"=w100, "控制命令"=w97) -> ("控制命令"=w104:u16[])  [unwired: 9 in]
        n68 = local read "站号"() -> (w103:u16)
        n69 = Bundle("站号"=w103, "控制命令"=w104) -> (w102:cluster{"站号":u16, "控制命令":u16[]})  [unwired: 1 in]
        n70 = Bundle By Name(cluster=cluster{"命令":string, "data":variant} {"命令"="", "data"=variant} ("元素"), "命令"="启动", "data"=w102) -> (w106:cluster{"命令":string, "data":variant})
        n71 = Enqueue Element(queue=w108, element=w106) -> ()  [unwired: 2 in, 3 out]
      }
      event "停止": Value Change {
        n72 = event-data() -> ()  [unwired: 1 in, 6 out]
        n73 = Set Occurrence(w115) -> ()
        n74 = Flush Queue(queue=w118) -> (queue out=w117:refnum<queue>)  [unwired: 1 in, 2 out]
        n75 = Enqueue Element(queue=w117, element=cluster{"命令":string, "data":variant} {"命令"="shutdown", "data"=variant} ("元素")) -> ()  [unwired: 2 in, 3 out]
      }
      event "读测量数据区": Value Change {
        n76 = event-data() -> ()  [unwired: 1 in, 6 out]
        n77 = Bundle By Name(cluster=cluster{"命令":string, "data":variant} {"命令"="", "data"=variant} ("元素"), "命令"="读测量数据区", "data"="站号") -> (w122:cluster{"命令":string, "data":variant})
        n78 = Enqueue Element(queue=w124, element=w122) -> ()  [unwired: 2 in, 3 out]
      }
      event "读状态告警区": Value Change {
        n79 = event-data() -> ()  [unwired: 1 in, 6 out]
        n80 = local read "站号"() -> (w125:u16)
        n81 = Bundle By Name(cluster=cluster{"命令":string, "data":variant} {"命令"="", "data"=variant} ("元素"), "命令"="读状态告警区", "data"=w125) -> (w127:cluster{"命令":string, "data":variant})
        n82 = Enqueue Element(queue=w129, element=w127) -> ()  [unwired: 2 in, 3 out]
      }
      event "读关键参数区": Value Change {
        n83 = event-data() -> ()  [unwired: 1 in, 6 out]
        n84 = local read "站号"() -> (w130:u16)
        n85 = Bundle By Name(cluster=cluster{"命令":string, "data":variant} {"命令"="", "data"=variant} ("元素"), "命令"="读关键参数区", "data"=w130) -> (w132:cluster{"命令":string, "data":variant})
        n86 = Enqueue Element(queue=w134, element=w132) -> ()  [unwired: 2 in, 3 out]
      }
    }
  }
  n87 = while {
    tunnel: w38 -> [w145]
    tunnel: w37 -> [w141]
    stop <- w142 stop-if-true
    n88 = global read "总磷总氮断电保存全局变量.vi" "MB通信方式选择"() -> (w140:enum16{"串口", "TCP"})
    n89 = Wait on Occurrence(2:w145, 3:10000 ("毫秒超时(-1)")) -> (0:w143:bool)  [unwired: 1 in]
    n90 = Not(x=w143) -> (.not. x?=w142:bool)
    n91 = case shown="\"TCP\"" w140 {
      tunnel: [_ w146] -> w137
      frame "串口", Default {
      }
      frame "TCP" {
        n92 = global read "VAR总磷总氮全局变量.vi" "MB session in"() -> (w148:refnum<class "MB_Master.lvclass">)
        n93 = property class="MB_Master"(reference=w148) -> ("Properties:Session Valid"=w147:bool)  [unwired: 1 in, 2 out]
        n94 = Not(x=w147) -> (.not. x?=w146:bool)
      }
    }
    n95 = First Call?() -> (First Call?: T/F=w139:bool)
    n96 = Or(x=w137, y=w139) -> (x .or. y?=w138:bool)
    n97 = local read "启用"() -> (w135:bool)
    n98 = And(x=w135, y=w138) -> (x .and. y?=w136:bool)
    n99 = case shown="True" w136 {
      tunnel: w141 -> [_ w151]
      frame False {
      }
      frame True {
        n100 = Flush Queue(queue=w151) -> (queue out=w149:refnum<queue>)  [unwired: 1 in, 2 out]
        n101 = Enqueue Element(queue=w149, element=cluster{"命令":string, "data":variant} {"命令"="启用模块", "data"=variant} ("元素")) -> ()  [unwired: 2 in, 3 out]
        n102 = property on="VISA Resource" class="VISAName"("DisabledEnum"=T15."Disabled and Grayed Out" ("禁用")) -> ()  [unwired: 2 in, 2 out]
      }
    }
  }
  n103 = while {
    tunnel: w37 -> [w169]
    tunnel: w40 -> [w168]
    shift-right: [w155] -> _
    shift-left: _ -> [w166]
    tunnel: errorcluster {"status"=FALSE, "code"=0, "source"=""} ("error out") -> [w165]
    tunnel: [w161] -> _
    stop <- w167 stop-if-true
    n104 = Dequeue Element(queue=w169, error in (no error)=w168) -> (queue out=w162:refnum<queue>, element=w163:cluster{"命令":string, "data":variant})  [unwired: 1 in, 2 out]
    n105 = Unbundle By Name(w163) -> ("命令"=w164:string, "data"=w159:variant)
    n106 = case shown="\"读状态告警区\"" w164 {
      tunnel: w159 -> [_ _ _ w206 w217 w234 w237 w353 w413 _]
      tunnel: w162 -> [_ _ _ _ _ _ w238 _ _ w426]
      tunnel: [_ _ _ _ _ _ _ _ _ TRUE] -> w167
      tunnel: [w172 w175 w193 w209 w220 w236 w264 w361 w420 w422] -> w155
      tunnel: [w173 w174 w194 w208 w219 w235 w265 w352 w421 w423] -> w161
      tunnel: w166 -> [w172 _ w193 w205 w216 w233 w260 w356 w416 w422]
      tunnel: w165 -> [w173 _ w195 w202 w213 w230 w258 w357 w417 w424]
      tunnel: [_ _ _ w197 w210 w224 w250 w335 w407 _] -> w153
      frame Default {
      }
      frame "启用模块" {
        n107 = global read "总磷总氮断电保存全局变量.vi" "MB通信方式选择"() -> (w176:enum16{"串口", "TCP"})
        n108 = case shown="\"串口\", Default" w176 {
          tunnel: [w184 w189] -> w174
          tunnel: [w181 w188] -> w175
          frame "串口", Default {
            n109 = global read "总磷总氮断电保存全局变量.vi" "波特率"() -> (w179:u32)
            n110 = global read "总磷总氮断电保存全局变量.vi" "VISA Resource"() -> (w182:refnum<visa-resource-name>)
            n111 = Bundle By Name(cluster=T16 {"baud rate (bps)"=115200, "stop bits"=10, "parity"=0, "flow control"=0, "timeout"=1000, "retries"=1} ("Serial Config"), "baud rate (bps)"=w179) -> (w178:T16)
            n112 = call <vilib>:"Open Serial Session.vi"("Mode (RTU)"=enum16{"RTU", "ASCII"}."RTU", "Slave ID"=u8 1, "Serial Config"=w178, "VISA Resource"=w182) -> ("Error out"=w184:errorcluster, "MB_Serial session"=w181:refnum<class "MB_Master_Serial.lvclass">)  [unwired: 6 in]
          }
          frame "TCP" {
            n113 = global read "总磷总氮断电保存全局变量.vi" "PORT"() -> (w187:string)
            n114 = Decimal String To Number(string=w187) -> (number=w190:i32)  [unwired: 2 in, 1 out]
            n115 = global read "总磷总氮断电保存全局变量.vi" "IP"() -> (w186:string)
            n116 = call <vilib>:"Open TCP Session.vi"("Port (502)"=w190, "IP Address"=w186) -> ("error out"=w189:errorcluster, "MB_TCP session"=w188:refnum<class "MB_Master_TCP.lvclass">)  [unwired: 8 in]
          }
        }
        "启用" <- TRUE
      }
      frame "停用模块" {
        n117 = call-dynamic "Close Session.vi"("error in (no error)"=w195, "MB session in"=w193) -> ("error out"=w191:errorcluster)  [unwired: 9 in]
        n118 = local write "启用"(FALSE ("启用")) -> ()
        n119 = call <vilib>:"Clear Errors.vi"("error in (no error)"=w191) -> ("error out"=w194:errorcluster)  [unwired: 5 in, 1 out]
      }
      frame "启动" {
        n120 = Variant To Data(type=cluster{"站号":u16, "控制命令":u16[]} {"站号"=0, "控制命令"=[]} ("输出簇"), Variant=w206) -> (data=w200:cluster{"站号":u16, "控制命令":u16[]})  [unwired: 1 in, 1 out]
        n121 = Unbundle By Name(w200) -> ("站号"=w197:u16, "控制命令"=w198:u16[])
        n122 = property class="MB_Master"(reference=w205, error in=w202, "Properties:Slave ID"=w197) -> (reference out=w204:refnum<class "MB_Master.lvclass">, error out=w203:errorcluster)
        n123 = Index Array(array=w198) -> (element=w199:u16)  [unwired: 1 in]
        n124 = Swap Bytes(anything=w199) -> (byte swapped=w196:u16)
        n125 = global write "VAR总磷总氮全局变量.vi" "控制命令"(w196) -> ()
        n126 = call <vilib>:"Write Multiple Registers.vi"("error in (no error)"=w203, "values"=w198, "starting address"=u16 4608, "MB session in"=w204) -> ("error out"=w208:errorcluster, "MB session out"=w209:refnum<class "MB_Master.lvclass">)  [unwired: 6 in]
      }
      frame "盲样测试" {
        n127 = Variant To Data(type=u8 0, Variant=w217) -> (data=w210:u8)  [unwired: 1 in, 1 out]
        n128 = property class="MB_Master"(reference=w216, error in=w213, "Properties:Slave ID"=w210) -> (reference out=w215:refnum<class "MB_Master.lvclass">, error out=w214:errorcluster)
        n129 = case shown="Default" w210 {
          tunnel: [u16[] [] ("values") u16[] [33539, 0] ("values") u16[] [23555, 0] ("values")] -> w212
          frame Default {
          }
          frame 1 {
            # "总磷盲样测试命令"
          }
          frame 3 {
            # "氨氮盲样测试"
          }
        }
        n130 = call <vilib>:"Write Multiple Registers.vi"("error in (no error)"=w214, "values"=w212, "starting address"=u16 24592, "MB session in"=w215) -> ("error out"=w219:errorcluster, "MB session out"=w220:refnum<class "MB_Master.lvclass">)  [unwired: 6 in]
      }
      frame "debug" {
        n131 = Variant To Data(type=cluster{"站号":u16, "控制命令":u16[]} {"站号"=0, "控制命令"=[]} ("输出簇"), Variant=w234) -> (data=w228:cluster{"站号":u16, "控制命令":u16[]})  [unwired: 1 in, 1 out]
        n132 = Unbundle By Name(w228) -> ("站号"=w224:u16, "控制命令"=w226:u16[])
        n133 = property class="MB_Master"(reference=w233, error in=w230, "Properties:Slave ID"=w224) -> (reference out=w232:refnum<class "MB_Master.lvclass">, error out=w231:errorcluster)
        n134 = Index Array(array=w226) -> (element=w227:u16)  [unwired: 1 in]
        n135 = global write "VAR总磷总氮全局变量.vi" "控制命令"(w227) -> ()
        n136 = call <vilib>:"Write Multiple Registers.vi"("error in (no error)"=w231, "values"=w226, "starting address"=u16 24594, "MB session in"=w232) -> ("error out"=w235:errorcluster, "MB session out"=w236:refnum<class "MB_Master.lvclass">)  [unwired: 6 in]
      }
      frame "读测量数据区" {
        n137 = Variant To Data(type=u8 1 ("Slave ID"), Variant=w237) -> (data=w250:u8)  [unwired: 1 in, 1 out]
        n138 = property class="MB_Master"(reference=w260, error in=w258, "Properties:Slave ID"=w250) -> (reference out=w259:refnum<class "MB_Master.lvclass">, error out=w257:errorcluster)
        n139 = global read "VAR总磷总氮全局变量.vi" "测量数据区数组"() -> (w254:T8)
        n140 = call "id参数转换.vi"("id"=w250) -> ("数组资源索引"=w249:i32)  [unwired: 9 in, 1 out]
        n141 = Bundle("命令"="读关键参数区", "data"=w237) -> (w239:cluster{"命令":string, "data":variant})  [unwired: 1 in]
        n142 = call <vilib>:"Read Holding Registers.vi"("error in (no error)"=w257, "quantity"=u16 107, "starting address"=u16 4096, "MB session in"=w259) -> ("error out"=w265:errorcluster, "Registers"=w256:u16[], "MB session out"=w264:refnum<class "MB_Master.lvclass">)  [unwired: 5 in]
        n143 = Enqueue Element(queue=w238, element=w239) -> ()  [unwired: 2 in, 3 out]
        n144 = call "id参数转换.vi"("id"=u16 2) -> ("数组资源索引"=w246:i32)  [unwired: 9 in, 1 out]
        n145 = call "id参数转换.vi"("id"=u16 3) -> ("数组资源索引"=w244:i32)  [unwired: 9 in, 1 out]
        n146 = Index Array(array=w254, index #1=w249, index #2=w246, index #3=w244) -> (element #1=w255:T5, element #2=w251:T5, element #3=w248:T5)
        n147 = call "测量数据区.vi"("数组"=w256) -> ("测量数据区"=w241:T5)  [unwired: 10 in]
        "测量数据区" <- w241
        n148 = global write "VAR总磷总氮全局变量.vi" "测量数据区"(w241) -> ()
        n149 = global read "工况数据接口全局.vi" "data"() -> (w243:T17)
        n150 = case shown="1" w250 {
          tunnel: w241 -> [w267 w274 w315 w323 w330]
          tunnel: w256 -> [_ w287 w316 w324 w331]
          tunnel: w255 -> [_ w280 _ _ _]
          tunnel: [w267 w282 w315 w323 w330] -> w253
          tunnel: w251 -> [_ w278 _ _ _]
          tunnel: w248 -> [_ w277 _ _ _]
          tunnel: w243 -> [w266 w275 w314 w322 w329]
          tunnel: [w266 w268 w303 w317 w328] -> w242
          tunnel: w241 -> [_ _ w313 w321 w327]
          frame 0, Default {
          }
          frame 1 {
            n151 = Unbundle By Name(w274) -> ("F0"=w273:sgl, "F1"=w272:sgl, "F2"=w271:sgl, "F3"=w270:sgl, "X值"=w269:sgl)
            n152 = Bundle By Name(cluster=w275, "data.TP.TP.F0"=w273, "data.TP.TP.F1"=w272, "data.TP.TP.F2"=w271, "data.TP.TP.F3"=w270, "data.TP.TP.X0"=w269) -> (w268:T17)
            n153 = global read "VAR总磷总氮全局变量.vi" "模块名称"() -> (w286:string)
            n154 = Search and Replace String(input string=w286, search string="总磷" ("搜索字符串")) -> (result string=w283:string, offset past replacement=w284:i32)  [unwired: 6 in, 2 out]
            n155 = case shown="Default" w284 {
              tunnel: w283 -> [_ w293]
              tunnel: [_ w290] -> w281
              tunnel: [_ w288] -> w279
              frame -1 {
              }
              frame Default {
                n156 = Search and Replace String(input string=w293, search string="总氮" ("搜索字符串")) -> (offset past replacement=w296:i32)  [unwired: 6 in, 3 out]
                n157 = Search and Replace String(input string=w293, search string="氨氮" ("搜索字符串")) -> (offset past replacement=w291:i32)  [unwired: 6 in, 3 out]
                n158 = Not Equal?(x=w296, y=-1) -> (x != y?=w288:bool)
                n159 = Not Equal?(x=w291, y=-1) -> (x != y?=w289:bool)
                n160 = Or(x=w289, y=w288) -> (x .or. y?=w290:bool)
              }
            }
            n161 = Select(t=w278, s=w279, f=w277) -> (s? t:f=w276:T5)
            n162 = case shown="True" w281 {
              tunnel: [w298 w302] -> w282
              tunnel: w280 -> [_ w301]
              tunnel: w276 -> [_ w300]
              tunnel: w274 -> [w298 w299]
              frame False {
              }
              frame True {
                # "启动总磷总氮时间自动对齐"
                n163 = call "数据时间对齐.vi"("待对齐时间"=w299, "对齐参考时间"=w300, "已对齐时间输入"=w301) -> ("已对齐时间输出"=w302:T5)  [unwired: 8 in]
              }
            }
            "总磷测量数据区" <- w287
          }
          frame 2 {
            n164 = Unbundle By Name(w313) -> ("F0"=w312:sgl, "F1"=w311:sgl, "F2"=w310:sgl, "F3"=w309:sgl, "F4"=w308:sgl, "F5"=w307:sgl, "F6"=w306:sgl, "F7"=w305:sgl, "X值"=w304:sgl)
            n165 = Bundle By Name(cluster=w314, "data.TN.TN.F0"=w312, "data.TN.TN.F1"=w311, "data.TN.TN.F2"=w310, "data.TN.TN.F3"=w309, "data.TN.TN.F4"=w308, "data.TN.TN.F5"=w307, "data.TN.TN.F6"=w306, "data.TN.TN.F7"=w305, "data.TN.TN.X0"=w304) -> (w303:T17)
            "总氮测量数据区" <- w316
          }
          frame 3 {
            n166 = Unbundle By Name(w321) -> ("F0"=w320:sgl, "F1"=w319:sgl, "X值"=w318:sgl)
            n167 = Bundle By Name(cluster=w322, "data.NH3.NH3.F0"=w320, "data.NH3.NH3.F1"=w319, "data.NH3.NH3.X0"=w318) -> (w317:T17)
            "氨氮测量数据区" <- w324
          }
          frame 22 {
            n168 = Unbundle By Name(w327) -> ("F0"=w326:sgl, "F1"=w325:sgl)
            n169 = Bundle By Name(cluster=w329, "data.CODCr.CODCr.F0"=w326, "data.CODCr.CODCr.F1"=w325) -> (w328:T17)
            "COD测量数据区" <- w331
          }
        }
        n170 = global write "工况数据接口全局.vi" "data"(w242) -> ()
        n171 = Replace Array Subset(array=w254, new element=w253, index=w249) -> (w252:T8)
        n172 = global write "VAR总磷总氮全局变量.vi" "测量数据区数组"(w252) -> ()
      }
      frame "读状态告警区" {
        n173 = Variant To Data(type=u8 1 ("Slave ID"), Variant=w353) -> (data=w335:u8)  [unwired: 1 in, 1 out]
        n174 = property class="MB_Master"(reference=w356, error in=w357, "Properties:Slave ID"=w335) -> (reference out=w355:refnum<class "MB_Master.lvclass">, error out=w354:errorcluster)
        n175 = call "id参数转换.vi"("id"=w335) -> ("数组资源索引"=w347:i32)  [unwired: 9 in, 1 out]
        n176 = call <vilib>:"Read Holding Registers.vi"("error in (no error)"=w354, "quantity"=u16 44, "starting address"=u16 4224, "MB session in"=w355) -> ("error out"=w352:errorcluster, "Registers"=w350:u16[], "MB session out"=w361:refnum<class "MB_Master.lvclass">)  [unwired: 5 in]
        n177 = global read "VAR总磷总氮全局变量.vi" "状态告警区数组"() -> (w349:T7)
        n178 = call "状态告警区.vi"("数组"=w350) -> ("状态告警区 2"=w334:T18, "状态告警区"=w336:T4)  [unwired: 9 in]
        n179 = Bundle By Name(cluster=w334, "id"=u16 22) -> (w332:T18)
        "状态告警区" <- w332
        n180 = global write "VAR总磷总氮全局变量.vi" "状态告警区"(w332) -> ()
        n181 = Unbundle By Name(w336) -> ("日志代码"=w337:u16, "告警代码"=w343:u16, "故障代码"=w341:u16)
        n182 = Unbundle By Name(w332) -> ("id"=w351:u16)
        n183 = Replace Array Subset(array=w349, new element=w336, index=w347) -> (w348:T7)
        n184 = global write "VAR总磷总氮全局变量.vi" "状态告警区数组"(w348) -> ()
        n185 = feedback-in #1(w343) -> ()
        n186 = feedback #1() -> (w344:u16)  [unwired: 1 in]
        n187 = feedback #2() -> (w342:u16)  [unwired: 1 in]
        n188 = feedback-in #2(w341) -> ()
        n189 = Not Equal?(x=w344, y=w343) -> (x != y?=w340:bool)
        n190 = Not Equal?(x=w342, y=w341) -> (x != y?=w339:bool)
        n191 = Or(x=w340, y=w339) -> (x .or. y?=w338:bool)
        n192 = global read "工况数据接口全局.vi" "data"() -> (w346:T17)
        n193 = case shown="22" w351 {
          tunnel: w336 -> [_ w374 w387 w397 w403]
          tunnel: w350 -> [_ w375 w388 w398 w405]
          tunnel: w346 -> [w362 w365 w380 w393 w404]
          tunnel: [w362 w372 w382 w396 w401] -> w345
          tunnel: w338 -> [_ w367 w378 w392 _]
          tunnel: w337 -> [_ w366 w377 w391 _]
          frame 0, Default {
          }
          frame 1, 131 {
            n194 = Unbundle By Name(w365) -> ("data.TP.TP.alarm_step"=w364:dbl)
            n195 = Unbundle By Name(w374) -> ("总磷控温温度1"=w373:sgl, "营养盐控温温度2"=w369:sgl)
            n196 = Select(t=w366, s=w367, f=w364) -> (s? t:f=w363:dbl)
            n197 = global read "VAR总磷总氮全局变量.vi" "总磷关键参数"() -> (w371:T19)
            n198 = Unbundle By Name(w371) -> ("消解温度"=w370:sgl)
            n199 = Bundle By Name(cluster=w365, "data.TP.TP.alarm_step"=w363, "data.TP.TP.digestion_temperature"=w373, "data.TP.TP.constant_temperature"=w370, "data.TP.TP.syringe_temperature"=w369, "data.TP.启用"=TRUE) -> (w372:T17)
            "总磷状态告警区" <- w375
          }
          frame 2, 76 {
            n200 = Unbundle By Name(w380) -> ("data.TN.TN.alarm_step"=w379:dbl)
            n201 = Unbundle By Name(w387) -> ("总磷控温温度1"=w383:sgl, "营养盐控温温度2"=w385:sgl)
            n202 = Select(t=w377, s=w378, f=w379) -> (s? t:f=w376:dbl)
            n203 = global read "VAR总磷总氮全局变量.vi" "总氮关键参数"() -> (w386:T19)
            n204 = Unbundle By Name(w386) -> ("消解温度"=w384:sgl)
            n205 = Bundle By Name(cluster=w380, "data.TN.TN.alarm_step"=w376, "data.TN.TN.digestion_temperature"=w383, "data.TN.TN.constant_temperature"=w384, "data.TN.TN.syringe_temperature"=w385, "data.TN.启用"=TRUE) -> (w382:T17)
            "总氮状态告警区" <- w388
          }
          frame 3 {
            n206 = Unbundle By Name(w393) -> ("data.NH3.NH3.alarm_step"=w390:dbl)
            n207 = Unbundle By Name(w397) -> ("营养盐控温温度2"=w395:sgl)
            n208 = Select(t=w391, s=w392, f=w390) -> (s? t:f=w389:dbl)
            n209 = Bundle By Name(cluster=w393, "data.NH3.NH3.alarm_step"=w389, "data.NH3.NH3.syringe_temperature"=w395, "data.NH3.启用"=TRUE) -> (w396:T17)
            "氨氮状态告警区" <- w398
          }
          frame 22 {
            n210 = Unbundle By Name(w403) -> ("营养盐控温温度2"=w402:sgl)
            n211 = global read "VAR总磷总氮全局变量.vi" "波形图-消解温度"() -> (w399:sgl[])
            n212 = Bundle By Name(cluster=w404, "data.CODCr.CODCr.temperature_curve"=w399, "data.CODCr.CODCr.reagent_sensor"=w402, "data.CODCr.启用"=TRUE) -> (w401:T17)
            "COD状态告警区" <- w405
          }
        }
        n213 = global write "工况数据接口全局.vi" "data"(w345) -> ()
      }
      frame "读关键参数区" {
        n214 = Variant To Data(type=u8 1 ("Slave ID"), Variant=w413) -> (data=w407:u8)  [unwired: 1 in, 1 out]
        n215 = property class="MB_Master"(reference=w416, error in=w417, "Properties:Slave ID"=w407) -> (reference out=w415:refnum<class "MB_Master.lvclass">, error out=w414:errorcluster)
        n216 = call "id参数转换.vi"("id"=w407) -> ("数组资源索引"=w406:i32)  [unwired: 9 in, 1 out]
        n217 = call <vilib>:"Read Holding Registers.vi"("error in (no error)"=w414, "quantity"=u16 56, "starting address"=u16 4256, "MB session in"=w415) -> ("error out"=w421:errorcluster, "Registers"=w411:u16[], "MB session out"=w420:refnum<class "MB_Master.lvclass">)  [unwired: 5 in]
        n218 = global read "VAR总磷总氮全局变量.vi" "关键参数区数组"() -> (w410:T6)
        n219 = call "关键参数区.vi"("数组"=w411) -> ("关键参数区"=w409:T3)  [unwired: 10 in]
        "关键参数区" <- w409
        n220 = global write "VAR总磷总氮全局变量.vi" "关键参数区"(w409) -> ()
        n221 = Replace Array Subset(array=w410, new element=w409, index=w406) -> (w408:T6)
        n222 = global write "VAR总磷总氮全局变量.vi" "关键参数区数组"(w408) -> ()
      }
      frame "shutdown" {
        n223 = call-dynamic "Close Session.vi"("error in (no error)"=w424, "MB session in"=w422) -> ("error out"=w423:errorcluster)  [unwired: 9 in]
        n224 = Flush Queue(queue=w426) -> (queue out=w425:refnum<queue>)  [unwired: 1 in, 2 out]
        n225 = Release Queue(queue=w425) -> ()  [unwired: 2 in, 3 out]
      }
    }
    n226 = global write "VAR总磷总氮全局变量.vi" "MB session in"(w155) -> ()
    n227 = Unbundle By Name(w161) -> ("status"=w158:bool)
    n228 = Not(x=w158) -> (.not. x?=w160:bool)
    "status" <- w160
    n229 = call <vilib>:"Boolean Crossing PtByPt.vi"("direction"=enum16{"either", "false-true", "true-false"}."false-true", "input"=w158) -> ("crossing"=w157:bool)  [unwired: 1 in]
    n230 = case shown="False" w157 {
      tunnel: [u16 0 ("告警代码") u16 999 ("告警代码")] -> w154
      frame False {
      }
      frame True {
      }
    }
    n231 = global write "VAR总磷总氮全局变量.vi" "通讯状态"(w160) -> ()
    n232 = call "告警码字段定义.vi"("id"=w153, "告警代码"=w154) -> ()  [unwired: 9 in, 1 out]
  }
  n233 = while {
    tunnel: w35 -> [w438]
    tunnel: w34 -> [w437]
    tunnel: w33 -> [w436]
    tunnel: w32 -> [w435]
    tunnel: w31 -> [w434]
    tunnel: w30 -> [w433]
    tunnel: w29 -> [w432]
    tunnel: w28 -> [w431]
    tunnel: w27 -> [w430]
    tunnel: w26 -> [w429]
    stop <- FALSE stop-if-true
    n234 = global read "model config var.vi" "启动队列名称"() -> (w441:cluster{"String":string, "Value":u16}[])
    n235 = Wait (ms)(milliseconds to wait=u32 1000 ("等待时间（毫秒）")) -> ()  [unwired: 1 out]
    n236 = global read "VAR总磷总氮全局变量.vi" "固件版本号"() -> (w428:string)
    n237 = for {
      tunnel: w441 -> [w454] mode=indexing
      tunnel: w438 -> [w452]
      tunnel: w437 -> [w451]
      tunnel: w436 -> [w450]
      tunnel: w435 -> [w449]
      tunnel: w434 -> [w448]
      tunnel: w433 -> [w447]
      tunnel: w432 -> [w446]
      tunnel: w431 -> [w445]
      tunnel: w430 -> [w444]
      tunnel: w429 -> [w443]
      tunnel: w428 -> [w442]
      n238 = Unbundle By Name(w454) -> ("Value"=w453:u16)
      n239 = case shown="1" w453 {
        tunnel: w452 -> [_ _ _ _ w541 _]
        tunnel: w451 -> [_ _ _ _ w540 _]
        tunnel: w450 -> [_ _ _ w520 _ _]
        tunnel: w449 -> [_ _ _ w519 _ _]
        tunnel: w448 -> [w457 _ _ _ _ _]
        tunnel: w447 -> [w456 _ _ _ _ _]
        tunnel: w446 -> [_ w478 _ _ _ _]
        tunnel: w445 -> [_ w477 _ _ _ _]
        tunnel: w444 -> [_ _ w499 _ _ _]
        tunnel: w443 -> [_ _ w498 _ _ _]
        tunnel: w442 -> [w455 w476 w497 w518 w539 _]
        frame 1 {
          n240 = Get Queue Status(queue=w457) -> (queue out=w460:refnum<queue>, # elements in queue=w459:i32)  [unwired: 2 in, 6 out]
          n241 = Equal To 0?(x=w459) -> (x = 0?=w458:bool)
          n242 = case shown="True" w458 {
            tunnel: w456 -> [_ w472]
            tunnel: w460 -> [_ w473]
            tunnel: w455 -> [_ w461]
            frame False {
            }
            frame True {
              w463 = u16 1 items=["总磷"=1, "总氮"=2, "氨氮"=3, "磷酸盐"=4, "硝氮"=5, "亚硝氮"=6, "硅酸盐"=7, "硫化物"=8, "CODCr"=22]
              n243 = Unbundle By Name(w472) -> ("关键参数"=w470:T20)
              n244 = global read "VAR总磷总氮全局变量.vi" "总磷关键参数"() -> (w471:T19)
              n245 = global read "VAR总磷总氮全局变量.vi" "状态告警区数组"() -> (w465:T7)
              n246 = global read "VAR总磷总氮全局变量.vi" "平台试剂余量百分比"() -> (w475:sgl)
              n247 = call "id参数转换.vi"("id"=w463) -> ("数组资源索引"=w464:i32)  [unwired: 9 in, 1 out]
              n248 = call "转换关键参数(子VI).vi"("参数"=w463, "总磷关键参数"=w471, "关键参数输入"=w470) -> ("关键参数输出"=w469:T20)  [unwired: 8 in]
              n249 = global read "VAR总磷总氮全局变量.vi" "总磷关键参数改变"() -> (w468:bool)
              n250 = global read "VAR总磷总氮全局变量.vi" "总磷校准信息改变"() -> (w466:bool)
              n251 = global read "VAR总磷总氮全局变量.vi" "总磷校准信息"() -> (w467:T21)
              n252 = Index Array(array=w465, index=w464) -> (element=w462:T4)
              n253 = Bundle By Name(cluster=w472, "状态告警区"=w462, "平台试剂余量百分比"=w475, "关键参数"=w469, "关键参数改变"=w468, "校准信息"=w467, "校准信息改变"=w466, "固件版本号"=w461) -> (w474:T11)
              n254 = Enqueue Element(queue=w473, element=w474) -> ()  [unwired: 2 in, 3 out]
            }
          }
        }
        frame 2 {
          n255 = Get Queue Status(queue=w478) -> (queue out=w481:refnum<queue>, # elements in queue=w480:i32)  [unwired: 2 in, 6 out]
          n256 = Equal To 0?(x=w480) -> (x = 0?=w479:bool)
          n257 = case shown="True" w479 {
            tunnel: w481 -> [_ w494]
            tunnel: w477 -> [_ w492]
            tunnel: w476 -> [_ w482]
            frame False {
            }
            frame True {
              w484 = u16 2 items=["总磷"=1, "总氮"=2, "氨氮"=3, "磷酸盐"=4, "硝氮"=5, "亚硝氮"=6, "硅酸盐"=7, "硫化物"=8, "CODCr"=22]
              n258 = Unbundle By Name(w492) -> ("关键参数"=w491:T20)
              n259 = global read "VAR总磷总氮全局变量.vi" "总氮关键参数"() -> (w493:T19)
              n260 = global read "VAR总磷总氮全局变量.vi" "状态告警区数组"() -> (w485:T7)
              n261 = global read "VAR总磷总氮全局变量.vi" "平台试剂余量百分比"() -> (w496:sgl)
              n262 = call "id参数转换.vi"("id"=w484) -> ("数组资源索引"=w486:i32)  [unwired: 9 in, 1 out]
              n263 = call "转换关键参数(子VI).vi"("参数"=w484, "总磷关键参数"=w493, "关键参数输入"=w491) -> ("关键参数输出"=w490:T20)  [unwired: 8 in]
              n264 = global read "VAR总磷总氮全局变量.vi" "总氮关键参数改变"() -> (w489:bool)
              n265 = global read "VAR总磷总氮全局变量.vi" "总氮校准信息改变"() -> (w487:bool)
              n266 = global read "VAR总磷总氮全局变量.vi" "总氮校准信息"() -> (w488:T21)
              n267 = Index Array(array=w485, index=w486) -> (element=w483:T4)
              n268 = Bundle By Name(cluster=w492, "状态告警区"=w483, "平台试剂余量百分比"=w496, "关键参数"=w490, "关键参数改变"=w489, "校准信息"=w488, "校准信息改变"=w487, "固件版本号"=w482) -> (w495:T12)
              n269 = Enqueue Element(queue=w494, element=w495) -> ()  [unwired: 2 in, 3 out]
            }
          }
        }
        frame 3 {
          (unwired) FALSE
          n270 = Get Queue Status(queue=w499) -> (queue out=w501:refnum<queue>, # elements in queue=w502:i32)  [unwired: 2 in, 6 out]
          n271 = Equal To 0?(x=w502) -> (x = 0?=w500:bool)
          n272 = case shown="True" w500 {
            tunnel: w501 -> [_ w515]
            tunnel: w498 -> [_ w514]
            tunnel: w497 -> [_ w503]
            frame False {
            }
            frame True {
              w505 = u16 3 items=["总磷"=1, "总氮"=2, "氨氮"=3, "磷酸盐"=4, "硝氮"=5, "亚硝氮"=6, "硅酸盐"=7, "硫化物"=8, "CODCr"=22]
              n273 = Unbundle By Name(w514) -> ("关键参数"=w513:T20)
              n274 = global read "VAR总磷总氮全局变量.vi" "氨氮关键参数"() -> (w511:T19)
              n275 = global read "VAR总磷总氮全局变量.vi" "状态告警区数组"() -> (w506:T7)
              n276 = global read "VAR总磷总氮全局变量.vi" "平台试剂余量百分比"() -> (w517:sgl)
              n277 = call "id参数转换.vi"("id"=w505) -> ("数组资源索引"=w507:i32)  [unwired: 9 in, 1 out]
              n278 = call "转换关键参数(子VI).vi"("参数"=w505, "总磷关键参数"=w511, "关键参数输入"=w513) -> ("关键参数输出"=w512:T20)  [unwired: 8 in]
              n279 = global read "VAR总磷总氮全局变量.vi" "氨氮关键参数改变"() -> (w510:bool)
              n280 = global read "VAR总磷总氮全局变量.vi" "氨氮校准信息改变"() -> (w508:bool)
              n281 = global read "VAR总磷总氮全局变量.vi" "氨氮校准信息"() -> (w509:T21)
              n282 = Index Array(array=w506, index=w507) -> (element=w504:T4)
              n283 = Bundle By Name(cluster=w514, "状态告警区"=w504, "平台试剂余量百分比"=w517, "关键参数"=w512, "关键参数改变"=w510, "校准信息"=w509, "校准信息改变"=w508, "固件版本号"=w503) -> (w516:T13)
              n284 = Enqueue Element(queue=w515, element=w516) -> ()  [unwired: 2 in, 3 out]
            }
          }
        }
        frame 22 {
          n285 = Get Queue Status(queue=w520) -> (queue out=w522:refnum<queue>, # elements in queue=w523:i32)  [unwired: 2 in, 6 out]
          n286 = Equal To 0?(x=w523) -> (x = 0?=w521:bool)
          n287 = case shown="True" w521 {
            tunnel: w522 -> [_ w536]
            tunnel: w519 -> [_ w535]
            tunnel: w518 -> [_ w524]
            frame False {
            }
            frame True {
              w526 = u16 22 items=["总磷"=1, "总氮"=2, "氨氮"=3, "磷酸盐"=4, "硝氮"=5, "亚硝氮"=6, "硅酸盐"=7, "硫化物"=8, "CODCr"=22]
              n288 = Unbundle By Name(w535) -> ("关键参数"=w534:T20)
              n289 = global read "VAR总磷总氮全局变量.vi" "CODcr关键参数"() -> (w533:T19)
              n290 = global read "VAR总磷总氮全局变量.vi" "状态告警区数组"() -> (w527:T7)
              n291 = global read "VAR总磷总氮全局变量.vi" "CODCr关键参数改变"() -> (w531:bool)
              n292 = global read "VAR总磷总氮全局变量.vi" "CODCr校准信息改变"() -> (w529:bool)
              n293 = global read "VAR总磷总氮全局变量.vi" "平台试剂余量百分比"() -> (w538:sgl)
              n294 = call "id参数转换.vi"("id"=w526) -> ("数组资源索引"=w528:i32)  [unwired: 9 in, 1 out]
              n295 = call "转换关键参数(子VI).vi"("参数"=w526, "总磷关键参数"=w533, "关键参数输入"=w534) -> ("关键参数输出"=w532:T20)  [unwired: 8 in]
              n296 = global read "VAR总磷总氮全局变量.vi" "CODCr校准信息"() -> (w530:T21)
              n297 = Index Array(array=w527, index=w528) -> (element=w525:T4)
              n298 = Bundle By Name(cluster=w535, "状态告警区"=w525, "平台试剂余量百分比"=w538, "关键参数"=w532, "关键参数改变"=w531, "校准信息"=w530, "校准信息改变"=w529, "固件版本号"=w524) -> (w537:T10)
              n299 = Enqueue Element(queue=w536, element=w537) -> ()  [unwired: 2 in, 3 out]
            }
          }
        }
        frame 21 {
          (unwired) FALSE
          n300 = Get Queue Status(queue=w541) -> (queue out=w543:refnum<queue>, # elements in queue=w544:i32)  [unwired: 2 in, 6 out]
          n301 = Equal To 0?(x=w544) -> (x = 0?=w542:bool)
          n302 = case shown="True" w542 {
            tunnel: w543 -> [_ w557]
            tunnel: w540 -> [_ w556]
            tunnel: w539 -> [_ w545]
            frame False {
            }
            frame True {
              w547 = u16 21 items=["总磷"=1, "总氮"=2, "氨氮"=3, "磷酸盐"=4, "硝氮"=5, "亚硝氮"=6, "硅酸盐"=7, "硫化物"=8, "CODMn"=21, "CODCr"=22, "氟化物"=50]
              n303 = Unbundle By Name(w556) -> ("关键参数"=w555:T20)
              n304 = global read "VAR总磷总氮全局变量.vi" "CODMn关键参数"() -> (w554:T19)
              n305 = global read "VAR总磷总氮全局变量.vi" "状态告警区数组"() -> (w548:T7)
              n306 = global read "VAR总磷总氮全局变量.vi" "CODmn关键参数改变"() -> (w552:bool)
              n307 = global read "VAR总磷总氮全局变量.vi" "CODMn校准信息改变"() -> (w550:bool)
              n308 = global read "VAR总磷总氮全局变量.vi" "平台试剂余量百分比"() -> (w559:sgl)
              n309 = call "id参数转换.vi"("id"=w547) -> ("数组资源索引"=w549:i32)  [unwired: 9 in, 1 out]
              n310 = call "转换关键参数(子VI).vi"("参数"=w547, "总磷关键参数"=w554, "关键参数输入"=w555) -> ("关键参数输出"=w553:T20)  [unwired: 8 in]
              n311 = global read "VAR总磷总氮全局变量.vi" "CODMn校准信息"() -> (w551:T21)
              n312 = Index Array(array=w548, index=w549) -> (element=w546:T4)
              n313 = Bundle By Name(cluster=w556, "状态告警区"=w546, "平台试剂余量百分比"=w559, "关键参数"=w553, "关键参数改变"=w552, "校准信息"=w551, "校准信息改变"=w550, "固件版本号"=w545) -> (w558:T10)
              n314 = Enqueue Element(queue=w557, element=w558) -> ()  [unwired: 2 in, 3 out]
            }
          }
        }
        frame Default {
        }
      }
    }
  }
  n315 = flat-sequence {
    tunnel: [w561] -> w8
    frame #0 {
      n316 = Wait (ms)(milliseconds to wait=u32 10000 ("等待时间（毫秒）")) -> ()  [unwired: 1 out]
    }
    frame #1 {
      n317 = global read "model config var.vi" "启动队列名称"() -> (w561:cluster{"String":string, "Value":u16}[])
    }
  }
  n318 = for {
    tunnel: w8 -> [w568] mode=indexing
    tunnel: [w563] -> w7 mode=indexing
    tunnel: [w562] -> w6 mode=indexing
    n319 = Unbundle By Name(w568) -> ("String"=w564:string)
    n320 = Concatenate Strings(w564, "固件升级" ("字符串")) -> (w566:string)
    n321 = Obtain Queue(name (unnamed)=w566, element data type=cluster{"selected path":path} {"selected path"=path ""}) -> (queue out=w563:refnum<queue>, error out=w562:errorcluster)  [unwired: 3 in, 1 out]
  }
  n322 = while {
    tunnel: w7 -> [w573]
    tunnel: w6 -> [w572]
    tunnel: [w571] -> _
    tunnel: [w570] -> _
    stop <- FALSE stop-if-true
    n323 = for {
      tunnel: w573 -> [w580] mode=indexing
      tunnel: w572 -> [w579] mode=indexing
      tunnel: [w578] -> w571
      tunnel: [w577] -> w570
      n324 = Dequeue Element(queue=w580, timeout in ms (-1)=1000 ("超时毫秒(-1)"), error in (no error)=w579) -> (queue out=w578:refnum<queue>, element=w576:cluster{"selected path":path}, timed out?=w574:bool, error out=w577:errorcluster)
      n325 = case shown="False" w574 {
        tunnel: w576 -> [w589 _]
        frame False {
          n326 = Unbundle By Name(w589) -> ("selected path"=w588:path)
          n327 = call "固件升级（包含参数恢复）.vi"("路径对话框"=FALSE, "selected path"=w588) -> ("结果字符串"=w582:string)  [unwired: 9 in]
          n328 = global read "VAR总磷总氮全局变量.vi" "模块名称"() -> (w584:string)
          n329 = Concatenate Strings("平台反控固件升级" ("日志信息"), w582) -> (w581:string)
          n330 = Get Date/Time In Seconds() -> (seconds since 1Jan1904=w585:timestamp)
          n331 = Bundle By Name(cluster=T22 {"时间"=timestamp(0 s since 1904-01-01), "参数"="", "日志信息"="", "流程参数"=""} ("data in"), "时间"=w585, "参数"=w584, "日志信息"=w581) -> (w586:T22)
          n332 = call "总磷总氮操作日志.vi"("data in"=w586) -> ()  [unwired: 10 in, 1 out]
        }
        frame True {
        }
      }
    }
  }
